vi "Autonomous Independent.vi"() -> ()   [LabVIEW 2013]
doc: "This VI is called when autonomous begins, and will automatically be terminated when autonomous ends. You can carry out timed or sensor driven robot movement independently without needing to return to the caller."
uses:
  Autonomous Setpoints.ctl
  Autonomous Center Line Setpoints.ctl
  Autonomous Commands.ctl
  Robot Global Data.vi
  <vilib>/Rock Robotics/WPI/RobotDrive/WPI_RobotDriveGetSetRefNum.vi
  <vilib>/Rock Robotics/WPI/RobotDrive/WPI_RobotDriveArcadeDrive_Standard(NoSaturation).vi
  <vilib>/addons/control/pid/pid.llb/PID (DBL).vi
  <vilib>/Rock Robotics/WPI/Joystick/WPI_JoystickGetSetRefNum.vi
  <vilib>/addons/control/pid/NI_PID_pid.lvlib
panel:
  out "Distance PID":T1
  out "Auto-Center Line":T2={"Arc Turn x-axis"=0.0, "Arc Turn y-axis"=0.8999999999999999, "Arc Turn Distance"=6.0, "Distance 1"=11.0, "Two Disc Distance 1"=0.0, "Distance 2"=-2.0, "Two Disc Distance 2"=0.0, "Spin Angle"=-70.0, "Spin Angle tolerance"=5.0, "Spin y-axis"=0.0, "Spin Distance"=0.0, "Center Line Enabled"=FALSE, "Distance 3"=8.5, "Two Disc Distance 3"=0.0, "Spin Angle 2"=90.0, "Spin Angle tolerance 2"=15.0, "Spin y-axis 2"=0.0, "Spin Distance 2"=0.0, "Shoot Angle 1"=14.6, "Disc Count 1"=4.0, "Shoot Time 1"=8000.0, "Shoot Angle 3"=16.4, "Disc Count 3"=5.0, "Shoot Time 3"=15000.0, "Low Gear"=TRUE}
  out "Auto Setpoints":T3={"Shoot Angle 1"=24.5, "Initial Delay"=0.0, "Disc Count 1"=3.0, "Shoot Time 1"=6000.0, "Distance 1"=6.5, "Two Disc Distance 1"=3.5, "Distance 2"=7.5, "Two Disc Distance 2"=3.5, "Distance 3"=-7.0, "Two Disc Distance 3"=0.0, "Shoot Angle 3"=31.0, "Disc Count 3"=4.0, "Shoot Time 3"=15000.0, "Distance 4"=0.0, "Two Disc Distance 4"=0.0, "Low Gear"=TRUE, "Shoot 1 Post Delay"=500.0}
  in  "Shoot Time 2":dbl
  in  "Disc Count 2":dbl
  in  "Shoot Angle 2":dbl
  out "Right Encoder":dbl(graph)
  out "Left Encoder":dbl(graph)
  out "Y axis Speed":dbl(graph)
  out "Steering":dbl(graph)
  out "Current Movement, for debugging":T4 {"Y Joystick Value" scale=1.0..-1.0; "X Joystick Value" scale=-1.0..1.0}
  in  "Array of robot movements":T5(array[cluster]) {"Y Joystick Value" scale=1.0..-1.0; "X Joystick Value" scale=-1.0..1.0}
  # "Be sure to right-click and choose Data Operations>>Make Current Value default if you want to save the array values with the VI"
  # "SKIP"
  # "SKIP"
  # "(Shoot 2 is not run)"
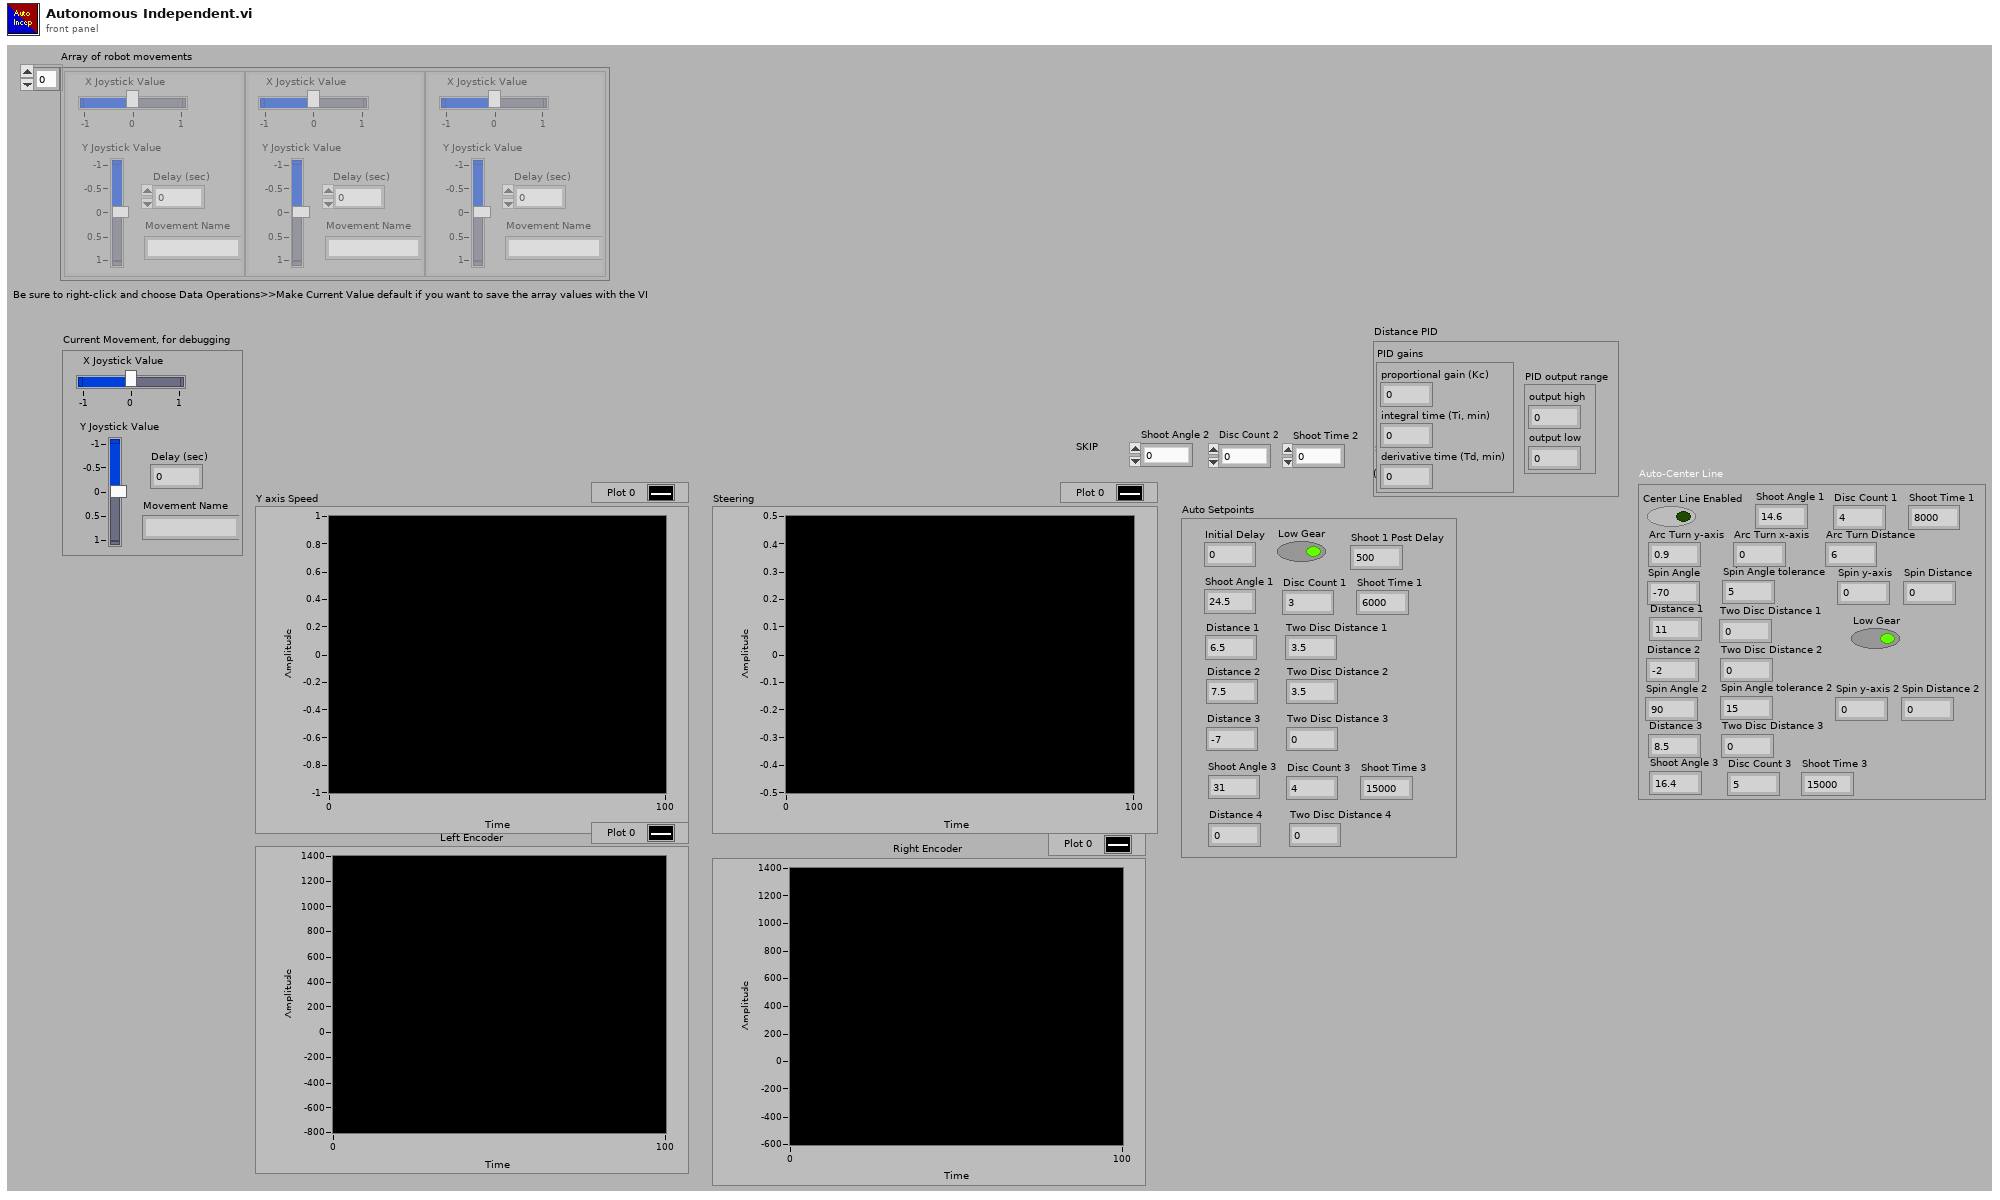
[diagram p1: front panel]
types:
  T1 = cluster{"PID gains":cluster{"proportional gain (Kc)":dbl, "integral time (Ti, min)":dbl, "derivative time (Td, min)":dbl}, "PID output range":cluster{"output high":dbl, "output low":dbl}}
  T2 = typedef "Autonomous Center Line Setpoints.ctl" = cluster{"Arc Turn x-axis":dbl, "Arc Turn y-axis":dbl, "Arc Turn Distance":dbl, "Distance 1":dbl, "Two Disc Distance 1":dbl, "Distance 2":dbl, "Two Disc Distance 2":dbl, "Spin Angle":dbl, "Spin Angle tolerance":dbl, "Spin y-axis":dbl, "Spin Distance":dbl, "Center Line Enabled":bool, "Distance 3":dbl, "Two Disc Distance 3":dbl, "Spin Angle 2":dbl, "Spin Angle tolerance 2":dbl, "Spin y-axis 2":dbl, "Spin Distance 2":dbl, "Shoot Angle 1":dbl, "Disc Count 1":dbl, "Shoot Time 1":dbl, "Shoot Angle 3":dbl, "Disc Count 3":dbl, "Shoot Time 3":dbl, "Low Gear":bool}
  T3 = typedef "Autonomous Setpoints.ctl" = cluster{"Shoot Angle 1":dbl, "Initial Delay":dbl, "Disc Count 1":dbl, "Shoot Time 1":dbl, "Distance 1":dbl, "Two Disc Distance 1":dbl, "Distance 2":dbl, "Two Disc Distance 2":dbl, "Distance 3":dbl, "Two Disc Distance 3":dbl, "Shoot Angle 3":dbl, "Disc Count 3":dbl, "Shoot Time 3":dbl, "Distance 4":dbl, "Two Disc Distance 4":dbl, "Low Gear":bool, "Shoot 1 Post Delay":dbl}
  T4 = cluster{"X Joystick Value":dbl, "Y Joystick Value":dbl, "Delay (sec)":dbl, "Movement Name":string}
  T5 = cluster{"X Joystick Value":dbl, "Y Joystick Value":dbl, "Delay (sec)":dbl, "Movement Name":string}[]
  T6 = typedef "Autonomous Commands.ctl" = cluster{"Load":bool, "Warmup":bool, "Low Gear":bool, "Shoot Angle":dbl, "Azimuth":bool, "Elevator":bool, "Neutral Angle":dbl, "Two Discs":bool, "Shoot":bool}
  T7 = typedef "WPI_RobotDriveDevRef.ctl" = cluster{"DevStatus":errorcluster, "Motors[]":T8[], "Square Inputs":bool, "Max Output":dbl, "Isochronous":bool}
  T8 = typedef "WPI_MotorControlDeviceRef.ctl" = cluster{"DeviceStatus":errorcluster, "Type":enum16{"PWM", "CAN"}, "PWM":cluster{"Digital Module":T9, "PWM Channel":T10, "DeadBand":T11}, "CAN":cluster{"Device Number":u8, "Control Mode":T12, "Semaphore":T13, "Max Vout":dbl}, "Invert":bool, "TransformRef":T14, "InvTransformRef":T14}
  T9 = typedef "FPGA_TypedefDigitalModule.ctl" = enum16{"Digital Module 1", "Digital Module 2"}
  T10 = typedef "FPGA_DIOPWMChannel.ctl" = enum8{"PWM 1", "PWM 2", "PWM 3", "PWM 4", "PWM 5", "PWM 6", "PWM 7", "PWM 8", "PWM 9", "PWM 10", "Invalid"}
  T11 = typedef "WPI_PWMDeadband.ctl" = cluster{"Name":string, "maxPositivePwm":i32, "minPositivePwm":i32, "centerPwm":i32, "maxNegativePwm":i32, "minNegativePwm":i32, "angularRange":u16}
  T12 = typedef "WPI_CANJaguar_ControlMode.ctl" = enum8{"Percent VBus", "Current", "Speed", "Position", "Voltage"}
  T13 = typedef "Semaphore RefNum" = refnum<k1>
  T14 = typedef "WPI_PWMTransform_ConPane.ctl" = refnum<vi>
  T15 = typedef "UDP Dashboard Packet.ctl" = cluster{"Feed Angle":dbl, "Neutral Angle":dbl, "Autonomous Setpoints":T3, "Auto Shift":T16, "Elevator Angle Offset":dbl, "Potentiometer Angle":cluster{"Pot M":dbl, "Pot B":dbl}, "Shoot Setpoints":cluster{"Vision":T17, "Back Corner":T17, "Front":T17, "Front Corner":T17, "Half Court":T17, "Full Court":T17, "Pyramid":T17}, "Halo Drive":T18, "Auto Speed Constants":T19, "Shooting Delays":cluster{"Unjam On":dbl, "Unjam Off":dbl, "Flipper On":dbl, "Flipper Off":dbl, "Hopper Up":dbl}, "Left Roller Pwr":dbl, "Right Roller Pwr":dbl, "Elevator PID Gains":cluster{"proportional gain (Kc)":dbl, "integral time (Ti, min)":dbl, "derivative time (Td, min)":dbl}, "Elevator PID Output Range":cluster{"output high":dbl, "output low":dbl}, "Elevator Angle Tolerance":dbl, "Toggle Ears Delay":dbl, "Toggle Ears Distance":dbl, "Unjam Servo Angle":dbl, "Auton Steer PID gains":cluster{"proportional gain (Kc)":dbl, "integral time (Ti, min)":dbl, "derivative time (Td, min)":dbl}, "Auton Steer output range":cluster{"output high":dbl, "output low":dbl}, "Auto Reverse Speed":dbl, "Auto Stop Throttle":dbl, "Auto Stop Duration":dbl, "Spin output range":cluster{"output high":dbl, "output low":dbl}, "Spin PID gains":cluster{"proportional gain (Kc)":dbl, "integral time (Ti, min)":dbl, "derivative time (Td, min)":dbl}, "Auto-Center Line":T2, "Auton Distance PID gains Low Gear":cluster{"proportional gain (Kc)":dbl, "integral time (Ti, min)":dbl, "derivative time (Td, min)":dbl}, "Auton Distance output range":cluster{"output high":dbl, "output low":dbl}, "Auton Distance Threshold":dbl, "Auton Velocity Cutoff":dbl, "Auton Distance output range Center Line":cluster{"output high":dbl, "output low":dbl}, "Auton Distance PID gains High Gear":cluster{"proportional gain (Kc)":dbl, "integral time (Ti, min)":dbl, "derivative time (Td, min)":dbl}}
  T16 = typedef "Auto Shift Settings.ctl" = cluster{"Enabled":bool, "Upshift Speed":dbl, "Downshift Speed":dbl, "Upshift Throttle":dbl, "Turn Power Diff":dbl, "Motor Limit":dbl, "Encoder Limit":dbl}
  T17 = typedef "Shoot Profile.ctl" = cluster{"Pre RPM":dbl, "Main RPM":dbl, "Angle":dbl}
  T18 = typedef "Halo Drive.ctl" = cluster{"Gains":cluster{"Quickturn_Sens_Low":dbl, "Quickturn_Sens_High":dbl, "Speedturn_Sens_Low":dbl, "Speedturn_Sens_High":dbl}, "QuickTurn Const":dbl, "Loading Throttle Limit":dbl}
  T19 = typedef "Auto Speed Constants.ctl" = cluster{"Slowing Distance":dbl, "High Speed":dbl, "Rampup Time":dbl, "Low Speed":dbl, "High Speed (Reverse)":dbl}
  T20 = cluster{"proportional gain (Kc)":dbl, "integral time (Ti, min)":dbl, "derivative time (Td, min)":dbl}
  T21 = typedef "WPI_GyroDevRef.ctl" = cluster{"DevStatus":errorcluster, "Analog Module":T22, "Analog Channel":T23, "Offset":dbl, "Gain (VoltsPerDegree/Second)":dbl}
  T22 = typedef "FPGA_TypedefAnalogModule.ctl" = enum16{"Analog Module 1", "Analog Module 2"}
  T23 = typedef "FPGA_AIChannel.ctl" = enum8{"AI 1", "AI 2", "AI 3", "AI 4", "AI 5", "AI 6", "AI 7", "AI 8", "Invalid"}
  T24 = typedef "WPI_JoystickDevRef.ctl" = cluster{"Device":T25}
  T25 = typedef "WPI_JoystickDeviceEnum.ctl" = enum16{"USB 1", "USB 2", "USB 3", "USB 4", "Kinect 1", "Kinect 2"}
  T26 = cluster{"axis 1 (x)":dbl, "axis 2 (y)":dbl, "axis 3 (throttle)":dbl, "axis 4":dbl, "axis 5":dbl, "axis 6":dbl}
  T27 = typedef "WPI_EncoderDevRef.ctl" = cluster{"DevStatus":errorcluster, "EncoderIndex":T28, "CounterIndex":T29, "DistancePerCount":dbl, "Decoding Type":T30}
  T28 = typedef "FPGA_EncoderIdx.ctl" = enum8{"Enc 0", "Enc 1", "Enc 2", "Enc 3", "Invalid"}
  T29 = typedef "FPGA_CounterCtrSystemIndex.ctl" = enum8{"Ctr 0", "Ctr 1", "Ctr 2", "Ctr 3", "Ctr 4", "Ctr 5", "Ctr 6", "Ctr 7", "Invalid"}
  T30 = typedef "WPI_EncoderType.ctl" = enum16{"1x", "2x", "4x"}
  T31 = typedef "Encoder Values.ctl" = cluster{"Left Dist":dbl, "Left Speed":dbl, "Right Dist":dbl, "Right Speed":dbl, "Left Ticks":dbl, "Right Ticks":dbl, "Avg Distance":dbl, "Avg Speed":dbl}
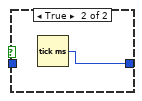
[diagram p3: hidden frame]
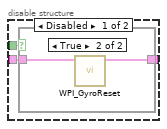
[diagram p4: hidden frame]
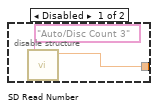
[diagram p6: hidden frame]
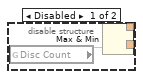
[diagram p7: hidden frame]
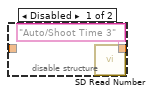
[diagram p8: hidden frame]
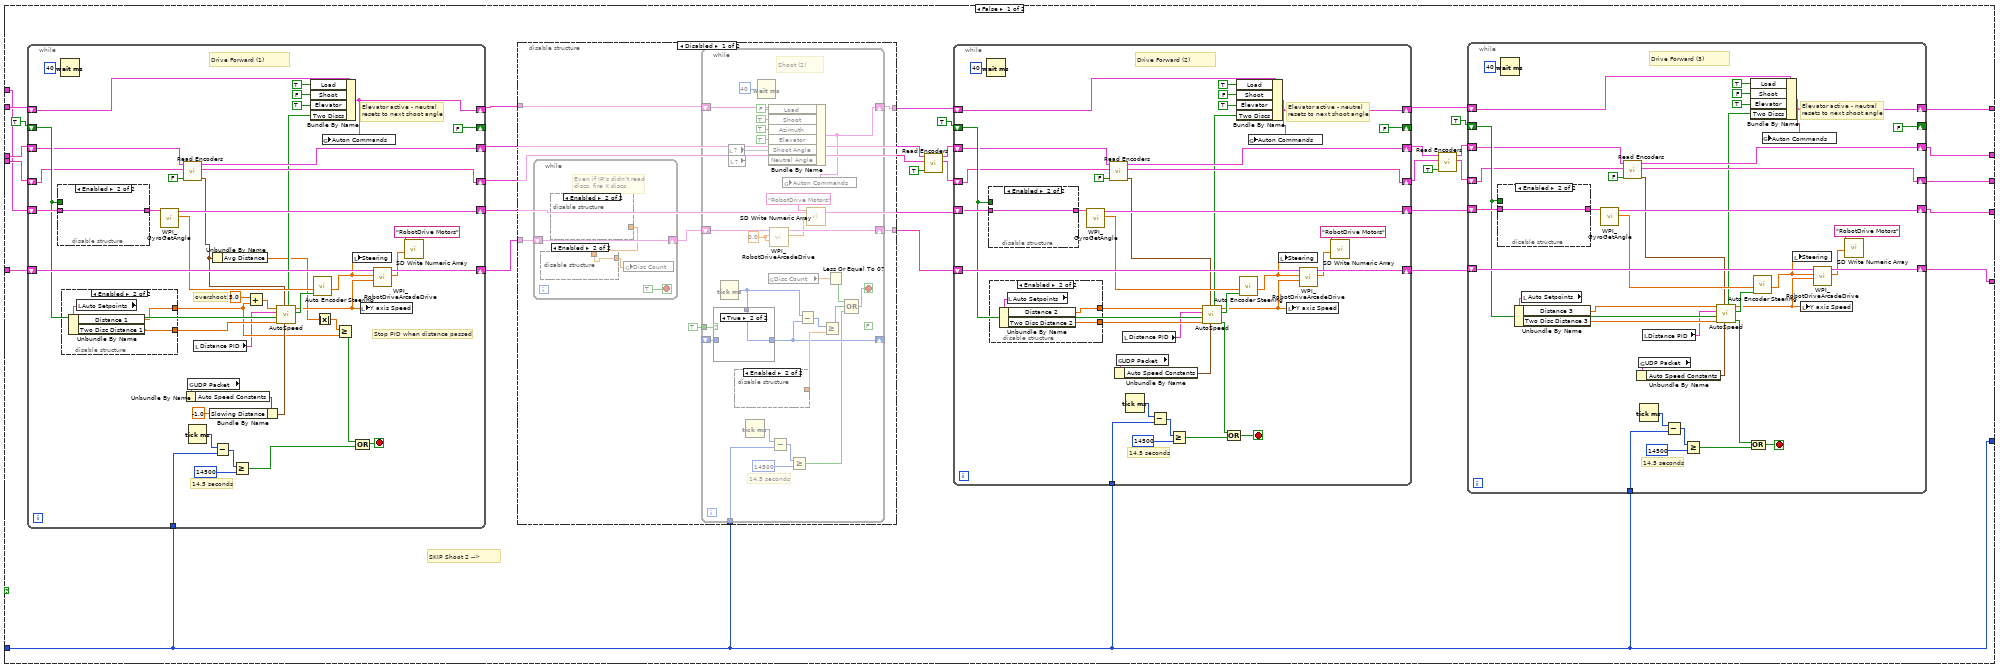
[diagram p10: hidden frame]
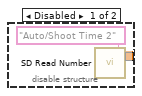
[diagram p11: hidden frame]
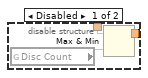
[diagram p13: hidden frame]
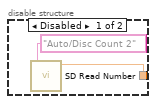
[diagram p14: hidden frame]
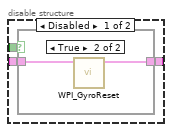
[diagram p16: hidden frame]
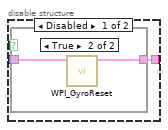
[diagram p18: hidden frame]
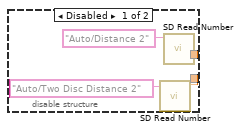
[diagram p20: hidden frame]
diagram:
  (unwired) "This code sets the toggle rate used by the Periodic Tasks VI.  For autonomous mode we slowly flash the USER1 LED on the cRIO.  Look at the Periodic Tasks VI to see how this global value is used."
  (unwired) "Autonomous sample code is disabled so your robot doesn't unexpectantly run in Autonomous mode.  To enable this code, right-click on the edge of the frame and choose either \"Remove Diagram Disable Structure\" or \"Enable This Subdiagram\". You should only enable one of the samples."
  (unwired) "This function is run in parallel when the autonomous period begins. It will be terminated automatically when the period ends.\n\nNote that all Driver Station inputs are automatically latched and will not change once auto begins."
  # "SKIP Shoot 2 -->"
  # "Every 20ms, report that we are running autonomous\ncode. Loop will abort the same time as the VI."
  # "Auton\nstart time"
  # "Auto\n\nShoot 3\n\nGo forward\nPick up center pyramid discs\nShoot 2\n\n\nPick up front pyramid discs\nGo back\nShoot 2"
  # "This gives you the joystick value\nthat is often the throttle"
  # "Use time and/or sensors to control how the robot drives."
  # "This tells you the driver position\nand alliance color"
  # "This gives you the eight Driver Station\ndigital switch settings"
  # "This gives you the four\nDriver Station sliders or\nanalog voltages"
  n1 = call <vilib>:"WPI_RobotDriveRefNum Registry Get.vi"("refnum name"="Left and Right Motors") -> ("RobotDriveDevRef"=w15:T7)  [unwired: 1 in, 9 out]
  n2 = while {
    tunnel: w15 -> [w47]
    tunnel: [w47] -> w14
    tunnel: [w44] -> w12
    tunnel: [w25] -> w4
    stop <- TRUE stop-if-true
    # "Replace Shoot 1 and 3 controls\nif in Center Line mode"
    n3 = global read "Robot Global Data.vi" "UDP Packet"() -> (w45:T15)
    n4 = Unbundle By Name(w45) -> ("Auton Distance PID gains Low Gear"=w30:T20, "Auton Distance PID gains High Gear"=w29:T20, "Auton Distance output range Center Line"=w26:cluster{"output high":dbl, "output low":dbl}, "Auton Distance output range"=w24:cluster{"output high":dbl, "output low":dbl}, "Autonomous Setpoints"=w43:T3, "Auto-Center Line"=w33:T2)
    "Auto-Center Line" <- w33
    n5 = Unbundle By Name(w33) -> ("Center Line Enabled"=w25:bool, "Shoot Angle 1"=w37:dbl, "Disc Count 1"=w38:dbl, "Shoot Time 1"=w39:dbl, "Shoot Angle 3"=w40:dbl, "Disc Count 3"=w41:dbl, "Shoot Time 3"=w42:dbl, "Low Gear"=w34:bool)
    n6 = Tick Count (ms)() -> (millisecond timer value=w44:u32)
    n7 = global write "Robot Global Data.vi" "Azimuth Ready"(TRUE ("Azimuth Ready")) -> ()
    n8 = case shown="True" w25 {
      tunnel: w43 -> [w49 w58]
      tunnel: [w49 w57] -> w32
      tunnel: w42 -> [_ w56]
      tunnel: w41 -> [_ w55]
      tunnel: w40 -> [_ w54]
      tunnel: w39 -> [_ w53]
      tunnel: w38 -> [_ w52]
      tunnel: w37 -> [_ w51]
      tunnel: w34 -> [_ w50]
      frame False {
      }
      frame True {
        n9 = Bundle By Name(cluster=w58, "Shoot Angle 1"=w51, "Disc Count 1"=w52, "Shoot Time 1"=w53, "Shoot Angle 3"=w54, "Disc Count 3"=w55, "Shoot Time 3"=w56, "Low Gear"=w50) -> (w57:T3)
      }
    }
    "Auto Setpoints" <- w32
    n10 = Unbundle By Name(w32) -> ("Low Gear"=w31:bool)
    n11 = Select(t=w30, s=w31, f=w29) -> (s? t:f=w28:T20)
    n12 = Select(t=w26, s=w25, f=w24) -> (s? t:f=w27:cluster{"output high":dbl, "output low":dbl})
    n13 = Bundle By Name(cluster=T1 {"PID gains"={"proportional gain (Kc)"=0.0, "integral time (Ti, min)"=0.0, "derivative time (Td, min)"=0.0}, "PID output range"={"output high"=0.0, "output low"=0.0}} ("Distance PID"), "PID gains"=w28, "PID output range"=w27) -> (→"Distance PID":T1)
  }
  n14 = while {
    stop <- FALSE stop-if-true
    n15 = call <vilib>:"WPI_DriverStationReport Robot Code State.vi"("Autonomous"=TRUE) -> ()  [unwired: 10 in, 1 out]
    n16 = Wait (ms)(milliseconds to wait=u32 20) -> ()  [unwired: 1 out]
  }
  n17 = disable-structure shown="Disabled" {
    frame Disabled {
      n18 = call <vilib>:"SD Read Number.vi"("Name"="Auto/Shoot Angle 1") -> ()  [unwired: 8 in, 3 out]
      n19 = call <vilib>:"SD Read Number.vi"("Name"="Auto/Shoot Angle 2") -> ()  [unwired: 8 in, 3 out]
      n20 = call <vilib>:"SD Read Number.vi"("Name"="Auto/Shoot Angle 3") -> ()  [unwired: 8 in, 3 out]
    }
    frame Enabled {
    }
  }
  n21 = global write "Robot Global Data.vi" "LED toggle rate (ms)"(u32 500 ("LED ms toggle rate")) -> ()
  n22 = disable-structure shown="Enabled" {
    frame Disabled {
      n23 = call <vilib>:"SD Read Boolean.vi"("Name"="Auto/Low Gear") -> ()  [unwired: 8 in, 3 out]
    }
    frame Enabled {
    }
  }
  n24 = while {
    tunnel: w14 -> [_]
    stop <- FALSE stop-if-true
    n25 = Wait (ms)(milliseconds to wait=u32 90) -> ()  [unwired: 1 out]
    n26 = call "Motor Output Report.vi"("Motor Speed"=0.0, "Motor refnum name"="Lift Motor 1" ("refnum name")) -> ()  [unwired: 9 in, 1 out]
  }
  n27 = call <vilib>:"WPI_DriverStationGet Alliance Info.vi"() -> ()  [unwired: 12 out]
  n28 = call <vilib>:"WPI_DriverStationGet Analog Input.vi"() -> ()  [unwired: 12 out]
  n29 = call <vilib>:"WPI_DriverStationGet Digital Input.vi"() -> ("Driver Station Digital Input (1-8)"=w23:bool[])  [unwired: 11 out]
  n30 = call <vilib>:"WPI_GyroRefNum Registry Get.vi"("refnum name"="Gyro") -> ("GyroDevRef"=w6:T21)  [unwired: 9 in, 1 out]
  n31 = while {
    shift-right: [w103] -> w11
    shift-left: w14 -> [w103]
    shift-right: [w100] -> _
    shift-left: _ -> [w99]
    shift-right: [FALSE] -> _
    shift-left: TRUE -> [w98]
    shift-right: [w95] -> w9
    shift-left: T6 {"Load"=FALSE, "Warmup"=FALSE, "Low Gear"=FALSE, "Shoot Angle"=35.0, "Azimuth"=FALSE, "Elevator"=FALSE, "Neutral Angle"=0.0, "Two Discs"=FALSE, "Shoot"=FALSE} ("Auton Commands") -> [w94]
    tunnel: w12 -> [w75]
    shift-right: [FALSE ("Load")] -> _
    shift-left: TRUE ("Elevator") -> [w74]
    shift-right: [w71] -> w5
    shift-left: w6 -> [w72]
    stop <- w77 stop-if-true
    # "14.5 seconds"
    # "Delay"
    # "Start with 3 Discs"
    n32 = local read "Auto Setpoints"() -> (w88:T3)
    n33 = Unbundle By Name(w88) -> ("Low Gear"=w85:bool, "Shoot Angle 1"=w87:dbl, "Shoot Angle 3"=w86:dbl, "Disc Count 1"=w84:dbl, "Initial Delay"=w82:dbl)
    n34 = case shown="True" w74 {
      tunnel: w72 -> [w104 w106]
      tunnel: [w104 w105] -> w71
      frame False {
      }
      frame True {
        n35 = call <vilib>:"WPI_GyroReset.vi"("GyroDevRef"=w106) -> ("GyroDevRef"=w105:T21)  [unwired: 9 in, 1 out]
      }
    }
    n36 = disable-structure shown="Enabled" {
      disable-tunnel: [w108 w109] -> w102
      disable-tunnel: w84 -> [_ w109]
      frame Disabled {
        n37 = call <vilib>:"SD Read Number.vi"("Name"="Auto/Disc Count 1") -> ("Numeric"=w108:dbl)  [unwired: 8 in, 2 out]
      }
      frame Enabled {
      }
    }
    n38 = Tick Count (ms)() -> (millisecond timer value=w96:u32)
    n39 = case shown="False" w98 {
      tunnel: [w113 w114] -> w100
      tunnel: w99 -> [w113 _]
      tunnel: w96 -> [_ w114]
      frame False {
      }
      frame True {
      }
    }
    n40 = disable-structure shown="Enabled" {
      disable-tunnel: [w110 w112] -> w83
      disable-tunnel: w82 -> [_ w112]
      frame Disabled {
        n41 = call <vilib>:"SD Read Number.vi"("Name"="Auto/Initial Delay") -> ("Numeric"=w110:dbl)  [unwired: 8 in, 2 out]
      }
      frame Enabled {
      }
    }
    n42 = Tick Count (ms)() -> (millisecond timer value=w81:u32)
    n43 = Subtract(x=w81, y=w75) -> (x-y=w80:u32)
    n44 = Greater Or Equal?(x=w80, y=u32 14500) -> (x >= y?=w76:bool)
    n45 = Bundle By Name(cluster=w94, "Load"=FALSE, "Shoot"=FALSE, "Low Gear"=w85, "Shoot Angle"=w87, "Azimuth"=FALSE, "Elevator"=TRUE, "Neutral Angle"=w86, "Two Discs"=FALSE, "Warmup"=FALSE) -> (w95:T6)
    n46 = global write "Robot Global Data.vi" "Auton Commands"(w95) -> ()
    n47 = Subtract(x=w96, y=w100) -> (x-y=w101:u32)
    n48 = global write "Robot Global Data.vi" "Disc Count"(w102) -> ()
    n49 = Greater Or Equal?(x=w101, y=w83) -> (x >= y?=w78:bool)
    n50 = Compound Arithmetic op=OR(w78, w76) -> (w77:bool)
  }
  n51 = call <vilib>:"WPI_JoystickRefNum Registry Get.vi"("refnum name"="Joystick 1") -> ("JoystickDevRef"=w21:T24)  [unwired: 1 in, 9 out]
  n52 = call <vilib>:"WPI_JoystickGet.vi"("JoystickDevRef"=w21) -> ("Axes"=w18:T26)  [unwired: 1 in, 5 out]
  n53 = Cluster To Array(cluster=w18) -> (array=w19:dbl[])
  n54 = Unbundle By Name(w18) -> ()  [unwired: 1 out]
  n55 = call <vilib>:"SD Write Numeric Array.vi"("Numeric Array"=w19, "Name"="Joystick 1/Axes") -> ()  [unwired: 8 in, 2 out]
  n56 = Index Array(array=w23) -> (element #1=w1:bool)  [unwired: 8 in, 7 out]
  n57 = disable-structure shown="Disabled" {
    frame Disabled {
      w115 = "RobotDrive Motors" ("Name")
      # "This is some simple sample code to drive your robot curving one direction and then the other."
      # "stand still"
      # "turn left for 0.5 second"
      # "turn right for 1 second"
      n58 = call <vilib>:"WPI_RobotDriveRefNum Registry Get.vi"("refnum name"="Left and Right Motors") -> ("RobotDriveDevRef"=w119:T7)  [unwired: 1 in, 9 out]
      n59 = call-poly <vilib>:"WPI_RobotDriveArcadeDrive.vi"("Y axis value"=0.5 ("X axis value"), "X axis value"=0.25, "RobotDriveDevRef"=w119) -> ("Motor Values"=w118:dbl[], "RobotDriveDevRef"=w126:T7)  [unwired: 1 in, 6 out]
      n60 = call <vilib>:"SD Write Numeric Array.vi"("Numeric Array"=w118, "Name"=w115) -> ()  [unwired: 8 in, 2 out]
      n61 = call <vilib>:"WPI_RobotDriveDelayAndUpdateSafety.vi"("Delay (s)"=1.0, "RobotDriveDevRef"=w126) -> ("RobotDriveDevRef 2"=w125:T7)  [unwired: 8 in, 1 out]
      n62 = call-poly <vilib>:"WPI_RobotDriveArcadeDrive.vi"("Y axis value"=0.25 ("X axis value"), "X axis value"=0.5, "RobotDriveDevRef"=w125) -> ("Motor Values"=w117:dbl[], "RobotDriveDevRef"=w124:T7)  [unwired: 1 in, 6 out]
      n63 = call <vilib>:"SD Write Numeric Array.vi"("Numeric Array"=w117, "Name"=w115) -> ()  [unwired: 8 in, 2 out]
      n64 = call <vilib>:"WPI_RobotDriveDelayAndUpdateSafety.vi"("Delay (s)"=0.5, "RobotDriveDevRef"=w124) -> ("RobotDriveDevRef 2"=w123:T7)  [unwired: 8 in, 1 out]
      n65 = call-poly <vilib>:"WPI_RobotDriveArcadeDrive.vi"("Y axis value"=0.0 ("X axis value"), "X axis value"=0.0, "RobotDriveDevRef"=w123) -> ("Motor Values"=w116:dbl[])  [unwired: 1 in, 7 out]
      n66 = call <vilib>:"SD Write Numeric Array.vi"("Numeric Array"=w116, "Name"=w115) -> ()  [unwired: 8 in, 2 out]
    }
    frame Enabled {
    }
  }
  n67 = disable-structure shown="Disabled" {
    frame Disabled {
      # "This sample code describes robot movements in an array. You can extend it to control other motors\non your robot. You can also use file I/O to move the data to a text file."
      n68 = call <vilib>:"WPI_RobotDriveRefNum Registry Get.vi"("refnum name"="Left and Right Motors") -> ("RobotDriveDevRef"=w134:T7)  [unwired: 1 in, 9 out]
      n69 = for {
        shift-right: [w140] -> _
        shift-left: w134 -> [w141]
        tunnel: "Array of robot movements" -> [w136] mode=indexing
        n70 = Unbundle By Name(w136) -> ("X Joystick Value"=w139:dbl, "Y Joystick Value"=w138:dbl, "Delay (sec)"=w137:dbl)  [unwired: 1 out]
        n71 = call-poly <vilib>:"WPI_RobotDriveArcadeDrive.vi"("Y axis value"=w138, "X axis value"=w139, "RobotDriveDevRef"=w141) -> ("Motor Values"=w143:dbl[], "RobotDriveDevRef"=w142:T7)  [unwired: 1 in, 6 out]
        n72 = call <vilib>:"SD Write Numeric Array.vi"("Numeric Array"=w143, "Name"="RobotDrive Motors") -> ()  [unwired: 8 in, 2 out]
        n73 = call <vilib>:"WPI_RobotDriveDelayAndUpdateSafety.vi"("Delay (s)"=w137, "RobotDriveDevRef"=w142) -> ("RobotDriveDevRef 2"=w140:T7)  [unwired: 8 in, 1 out]
        "Current Movement, for debugging" <- w136
      }
    }
    frame Enabled {
    }
  }
  n74 = case shown="False" w1 {
    tunnel: w12 -> [w146 w887]
    tunnel: w11 -> [w178 w906]
    tunnel: w9 -> [w175 w898]
    tunnel: w5 -> [w169 w897]
    tunnel: w4 -> [w154 _]
    tunnel: [w150 w892] -> w3
    tunnel: [w149 w893] -> w2
    frame False {
      # "Stop from coasting backwards"
      # "SKIP Shoot 2 -->"
      n75 = while {
        shift-right: [w873] -> w148
        shift-left: w178 -> [w874]
        shift-right: [w862] -> w177
        shift-left: w175 -> [w863]
        shift-right: [FALSE] -> _
        shift-left: TRUE -> [w857]
        shift-right: [w858] -> _
        shift-left: _ -> [w859]
        tunnel: w146 -> [w846]
        shift-right: [w842] -> w168
        shift-left: w169 -> [w842]
        stop <- w843 stop-if-true
        w871 = 0.0 ("Y axis value")
        # "14.5 seconds"
        # "Shoot (1)"
        n76 = local read "Auto Setpoints"() -> (w854:T3)
        n77 = Unbundle By Name(w854) -> ("Shoot Angle 1"=w853:dbl, "Shoot Angle 3"=w852:dbl, "Shoot Time 1"=w851:dbl)
        n78 = Tick Count (ms)() -> (millisecond timer value=w855:u32)
        n79 = case shown="True" w857 {
          tunnel: [w878 w879] -> w858
          tunnel: w859 -> [w878 _]
          tunnel: w855 -> [_ w879]
          frame False {
          }
          frame True {
          }
        }
        n80 = Wait (ms)(milliseconds to wait=u32 40) -> ()  [unwired: 1 out]
        n81 = disable-structure shown="Enabled" {
          disable-tunnel: [w875 w877] -> w856
          disable-tunnel: w851 -> [_ w877]
          frame Disabled {
            n82 = call <vilib>:"SD Read Number.vi"("Name"="Auto/Shoot Time 1") -> ("Numeric"=w875:dbl)  [unwired: 8 in, 2 out]
          }
          frame Enabled {
          }
        }
        n83 = Tick Count (ms)() -> (millisecond timer value=w847:u32)
        n84 = global read "Robot Global Data.vi" "Disc Count"() -> (w869:dbl)
        n85 = Subtract(x=w847, y=w846) -> (x-y=w848:u32)
        n86 = call-poly <vilib>:"WPI_RobotDriveArcadeDrive.vi"("Y axis value"=w871, "X axis value"=w871, "RobotDriveDevRef"=w874) -> ("Motor Values"=w872:dbl[], "RobotDriveDevRef"=w873:T7)  [unwired: 1 in, 6 out]
        n87 = Greater Or Equal?(x=w848, y=u32 14500) -> (x >= y?=w850:bool)
        n88 = Subtract(x=w855, y=w858) -> (x-y=w860:u32)
        n89 = call <vilib>:"SD Write Numeric Array.vi"("Numeric Array"=w872, "Name"="RobotDrive Motors") -> ()  [unwired: 8 in, 2 out]
        n90 = Bundle By Name(cluster=w863, "Load"=FALSE, "Shoot"=TRUE, "Azimuth"=FALSE, "Elevator"=TRUE, "Shoot Angle"=w853, "Neutral Angle"=w852) -> (w862:T6)
        n91 = global write "Robot Global Data.vi" "Auton Commands"(w862) -> ()
        n92 = Less Or Equal To 0?(x=w869) -> (x <= 0?=w844:bool)
        n93 = Greater Or Equal?(x=w860, y=w856) -> (x >= y?=w845:bool)
        n94 = Compound Arithmetic op=OR(w844, w845, w850) -> (w843:bool)
      }
      n95 = while {
        shift-right: [w196] -> w147
        shift-left: w148 -> [w197]
        tunnel: w146 -> [w190]
        shift-right: [FALSE] -> _
        shift-left: TRUE -> [w187]
        shift-right: [w185] -> _
        shift-left: _ -> [w184]
        stop <- w191 stop-if-true
        w198 = 0.0 ("Y axis value")
        # "Delay - after Shoot 1"
        # "14.5 seconds"
        n96 = local read "Auto Setpoints"() -> (w183:T3)
        n97 = Unbundle By Name(w183) -> ("Shoot 1 Post Delay"=w182:dbl)
        n98 = Tick Count (ms)() -> (millisecond timer value=w189:u32)
        n99 = case shown="True" w187 {
          tunnel: [w199 w200] -> w185
          tunnel: w184 -> [w199 _]
          tunnel: w189 -> [_ w200]
          frame False {
          }
          frame True {
          }
        }
        n100 = Tick Count (ms)() -> (millisecond timer value=w195:u32)
        n101 = Subtract(x=w195, y=w190) -> (x-y=w194:u32)
        n102 = Greater Or Equal?(x=w194, y=u32 14500) -> (x >= y?=w192:bool)
        n103 = Subtract(x=w189, y=w185) -> (x-y=w188:u32)
        n104 = Greater Or Equal?(x=w188, y=w182) -> (x >= y?=w181:bool)
        n105 = Compound Arithmetic op=OR(w181, w192) -> (w191:bool)
        n106 = call-poly <vilib>:"WPI_RobotDriveArcadeDrive.vi"("Y axis value"=w198, "X axis value"=w198, "RobotDriveDevRef"=w197) -> ("RobotDriveDevRef"=w196:T7)  [unwired: 1 in, 7 out]
      }
      n107 = call <vilib>:"WPI_EncoderRefNum Registry Get.vi"("refnum name"="Drive Encoder Left") -> ("EncoderDevRef"=w173:T27)  [unwired: 9 in, 1 out]
      n108 = call <vilib>:"WPI_EncoderRefNum Registry Get.vi"("refnum name"="Drive Encoder Right") -> ("EncoderDevRef"=w172:T27)  [unwired: 9 in, 1 out]
      n109 = call "Read Encoders.vi"("Reset"=TRUE, "Right Encoder"=w172, "Left Encoder"=w173) -> ("Right Encoder Out"=w170:T27, "Left Encoder Out"=w171:T27)  [unwired: 6 in, 1 out]
      n110 = case shown="True" w154 {
        tunnel: w146 -> [w310 w559]
        tunnel: w147 -> [w340 w605]
        tunnel: w177 -> [w339 w609]
        tunnel: w171 -> [w338 w608]
        tunnel: w170 -> [w337 w607]
        tunnel: w168 -> [w316 w606]
        tunnel: [w315 w576] -> w158
        tunnel: [w314 w575] -> w151
        tunnel: [w313 w574] -> w157
        tunnel: [w311 w572] -> w152
        tunnel: [w312 w573] -> w156
        tunnel: [w310 w559] -> w155
        frame False {
          # "SKIP Shoot 2 -->"
          n111 = while {
            shift-right: [w533] -> w320
            shift-left: w340 -> [w534]
            shift-right: [FALSE] -> _
            shift-left: TRUE -> [w518]
            shift-right: [w519] -> w318
            shift-left: w337 -> [w516]
            shift-right: [w520] -> w319
            shift-left: w338 -> [w517]
            shift-right: [w514] -> w317
            shift-left: w316 -> [w529]
            shift-right: [w521] -> w323
            shift-left: w339 -> [w522]
            tunnel: w310 -> [w505]
            stop <- w504 stop-if-true
            # "overshoot"
            # "Stop PID when distance passed"
            # "14.5 seconds"
            # "Elevator active - neutral\nresets to next shoot angle"
            # "Drive Forward (1)"
            n112 = disable-structure shown="Enabled" {
              disable-tunnel: w529 -> [w538 w542]
              disable-tunnel: w518 -> [w537 _]
              disable-tunnel: [w536 w542] -> w515
              frame Disabled {
                n113 = case shown="True" w537 {
                  tunnel: w538 -> [w539 w541]
                  tunnel: [w539 w540] -> w536
                  frame False {
                  }
                  frame True {
                    n114 = call <vilib>:"WPI_GyroReset.vi"("GyroDevRef"=w541) -> ("GyroDevRef"=w540:T21)  [unwired: 9 in, 1 out]
                  }
                }
              }
              frame Enabled {
              }
            }
            n115 = Wait (ms)(milliseconds to wait=u32 40) -> ()  [unwired: 1 out]
            n116 = disable-structure shown="Enabled" {
              disable-tunnel: [w545 w548] -> w496
              disable-tunnel: [w543 w547] -> w511
              frame Disabled {
                n117 = call <vilib>:"SD Read Number.vi"("Name"="Auto/Two Disc Distance 1") -> ("Numeric"=w543:dbl)  [unwired: 8 in, 2 out]
                n118 = call <vilib>:"SD Read Number.vi"("Name"="Auto/Distance 1") -> ("Numeric"=w545:dbl)  [unwired: 8 in, 2 out]
              }
              frame Enabled {
                n119 = local read "Auto Setpoints"() -> (w549:T3)
                n120 = Unbundle By Name(w549) -> ("Distance 1"=w548:dbl, "Two Disc Distance 1"=w547:dbl)
              }
            }
            n121 = call <vilib>:"WPI_GyroGetAngle.vi"("GyroDevRef"=w515) -> ("Angle"=w513:dbl, "GyroDevRef"=w514:T21)  [unwired: 7 in, 2 out]
            n122 = call "Read Encoders.vi"("Reset"=FALSE, "Right Encoder"=w516, "Left Encoder"=w517) -> ("Encoder Values"=w493:T31, "Right Encoder Out"=w519:T27, "Left Encoder Out"=w520:T27)  [unwired: 6 in]
            n123 = global read "Robot Global Data.vi" "UDP Packet"() -> (w503:T15)
            n124 = Unbundle By Name(w503) -> ("Auto Speed Constants"=w502:T19)
            n125 = Tick Count (ms)() -> (millisecond timer value=w506:u32)
            n126 = local read "Distance PID"() -> (w492:T1)
            n127 = Bundle By Name(cluster=w502, "Slowing Distance"=-1.0) -> (w500:T19)
            n128 = Unbundle By Name(w493) -> ("Avg Distance"=w494:dbl)
            n129 = Subtract(x=w506, y=w505) -> (x-y=w507:u32)
            n130 = Greater Or Equal?(x=w507, y=u32 14500) -> (x >= y?=w509:bool)
            n131 = Add(x=5.0, y=w496) -> (x+y=w498:dbl)
            n132 = call "AutoSpeed.vi"("Auto Speed Constants"=w500, "Encoder Values"=w493, "Two Disc Distance"=w511, "Reinitialize"=w518, "PID settings"=w492, "Target Distance"=w498) -> ("Backward"=w528:bool, "Y axis Speed"=w527:dbl, "Two Disc Loading"=w510:bool)  [unwired: 2 in, 1 out]
            n133 = Bundle By Name(cluster=w522, "Load"=TRUE, "Shoot"=FALSE, "Elevator"=TRUE, "Two Discs"=w510) -> (w521:T6)
            n134 = call "Auto Encoder Steering.vi"("Backward"=w528, "Gyro Angle"=w513) -> ("Steering"=w526:dbl)  [unwired: 8 in, 1 out]
            n135 = Absolute Value(x=w494) -> (abs(x)=w495:dbl)
            n136 = global write "Robot Global Data.vi" "Auton Commands"(w521) -> ()
            n137 = Greater Or Equal?(x=w495, y=w496) -> (x >= y?=w497:bool)
            n138 = local write "Steering"(w526) -> ()
            n139 = Compound Arithmetic op=OR(w497, w509) -> (w504:bool)
            n140 = local write "Y axis Speed"(w527) -> ()
            n141 = call-poly <vilib>:"WPI_RobotDriveArcadeDrive.vi"("Y axis value"=w527, "X axis value"=w526, "RobotDriveDevRef"=w534) -> ("Motor Values"=w532:dbl[], "RobotDriveDevRef"=w533:T7)  [unwired: 1 in, 6 out]
            n142 = call <vilib>:"SD Write Numeric Array.vi"("Numeric Array"=w532, "Name"="RobotDrive Motors") -> ()  [unwired: 8 in, 2 out]
          }
          n143 = disable-structure shown="Disabled" {
            disable-tunnel: w323 -> [w347 w393]
            disable-tunnel: [w346 w393] -> w322
            disable-tunnel: [w345 w392] -> w321
            disable-tunnel: w320 -> [w344 w392]
            disable-tunnel: w310 -> [w342 _]
            frame Disabled {
              n144 = while {
                shift-right: [w383] -> w348
                shift-left: w344 -> [w383]
                stop <- TRUE stop-if-true
                # "Even if IR's didn't read\ndiscs, fire X discs"
                n145 = disable-structure shown="Enabled" {
                  disable-tunnel: [w391 _] -> w382
                  frame Disabled {
                    n146 = call <vilib>:"SD Read Number.vi"("Name"="Auto/Disc Count 2") -> ("Numeric"=w391:dbl)  [unwired: 8 in, 2 out]
                  }
                  frame Enabled {
                  }
                }
                n147 = disable-structure shown="Enabled" {
                  disable-tunnel: [w387 w389] -> w384
                  disable-tunnel: w382 -> [w386 w389]
                  frame Disabled {
                    n148 = global read "Robot Global Data.vi" "Disc Count"() -> (w388:dbl)
                    n149 = Max & Min(x=w386, y=w388) -> (max(x,y)=w387:dbl)  [unwired: 1 out]
                  }
                  frame Enabled {
                  }
                }
                n150 = global write "Robot Global Data.vi" "Disc Count"(w384) -> ()
              }
              n151 = while {
                shift-right: [w376] -> w345
                shift-left: w348 -> [w377]
                shift-right: [w359] -> w346
                shift-left: w347 -> [w366]
                tunnel: TRUE -> [w363]
                shift-right: [w362] -> _
                shift-left: _ -> [w361]
                tunnel: w342 -> [w352]
                stop <- w349 stop-if-true
                (unwired) FALSE
                w374 = 0.0 ("Y axis value")
                # "14.5 seconds"
                # "Shoot (2)"
                n152 = Tick Count (ms)() -> (millisecond timer value=w360:u32)
                n153 = case shown="True" w363 {
                  tunnel: [w380 w381] -> w362
                  tunnel: w361 -> [w380 _]
                  tunnel: w360 -> [_ w381]
                  frame False {
                  }
                  frame True {
                  }
                }
                n154 = local read item#-1() -> (w358)
                n155 = local read item#-1() -> (w357)
                n156 = disable-structure shown="Enabled" {
                  disable-tunnel: [w378 _] -> w364
                  frame Disabled {
                    n157 = call <vilib>:"SD Read Number.vi"("Name"="Auto/Shoot Time 2") -> ("Numeric"=w378:dbl)  [unwired: 8 in, 2 out]
                  }
                  frame Enabled {
                  }
                }
                n158 = Tick Count (ms)() -> (millisecond timer value=w356:u32)
                n159 = Wait (ms)(milliseconds to wait=u32 40) -> ()  [unwired: 1 out]
                n160 = global read "Robot Global Data.vi" "Disc Count"() -> (w372:dbl)
                n161 = Bundle By Name(cluster=w366, "Load"=FALSE, "Shoot"=TRUE, "Azimuth"=TRUE, "Elevator"=TRUE, "Shoot Angle"=w358, "Neutral Angle"=w357) -> (w359:T6)
                n162 = call-poly <vilib>:"WPI_RobotDriveArcadeDrive.vi"("Y axis value"=w374, "X axis value"=w374, "RobotDriveDevRef"=w377) -> ("Motor Values"=w375:dbl[], "RobotDriveDevRef"=w376:T7)  [unwired: 1 in, 6 out]
                n163 = Subtract(x=w356, y=w352) -> (x-y=w355:u32)
                n164 = global write "Robot Global Data.vi" "Auton Commands"(w359) -> ()
                n165 = Greater Or Equal?(x=w355, y=u32 14500) -> (x >= y?=w353:bool)
                n166 = Subtract(x=w360, y=w362) -> (x-y=w365:u32)
                n167 = call <vilib>:"SD Write Numeric Array.vi"("Numeric Array"=w375, "Name"="RobotDrive Motors") -> ()  [unwired: 8 in, 2 out]
                n168 = Greater Or Equal?(x=w365, y=w364) -> (x >= y?=w351:bool)
                n169 = Less Or Equal To 0?(x=w372) -> (x <= 0?=w350:bool)
                n170 = Compound Arithmetic op=OR(w350, w351, w353) -> (w349:bool)
              }
            }
            frame Enabled {
            }
          }
          n171 = call "Read Encoders.vi"("Reset"=TRUE, "Right Encoder"=w318, "Left Encoder"=w319) -> ("Right Encoder Out"=w336:T27, "Left Encoder Out"=w335:T27)  [unwired: 6 in, 1 out]
          n172 = while {
            shift-right: [w475] -> w328
            shift-left: w321 -> [w476]
            shift-right: [FALSE] -> _
            shift-left: TRUE -> [w461]
            shift-right: [w462] -> w326
            shift-left: w336 -> [w459]
            shift-right: [w463] -> w325
            shift-left: w335 -> [w460]
            shift-right: [w457] -> w327
            shift-left: w317 -> [w471]
            shift-right: [w451] -> w324
            shift-left: w322 -> [w452]
            tunnel: w310 -> [w446]
            stop <- w444 stop-if-true
            # "14.5 seconds"
            # "Elevator active - neutral\nresets to next shoot angle"
            # "Drive Forward (2)"
            n173 = Wait (ms)(milliseconds to wait=u32 40) -> ()  [unwired: 1 out]
            n174 = disable-structure shown="Enabled" {
              disable-tunnel: w471 -> [w480 w484]
              disable-tunnel: w461 -> [w479 _]
              disable-tunnel: [w478 w484] -> w458
              frame Disabled {
                n175 = case shown="True" w479 {
                  tunnel: w480 -> [w481 w483]
                  tunnel: [w481 w482] -> w478
                  frame False {
                  }
                  frame True {
                    n176 = call <vilib>:"WPI_GyroReset.vi"("GyroDevRef"=w483) -> ("GyroDevRef"=w482:T21)  [unwired: 9 in, 1 out]
                  }
                }
              }
              frame Enabled {
              }
            }
            n177 = disable-structure shown="Enabled" {
              disable-tunnel: [w487 w490] -> w464
              disable-tunnel: [w485 w489] -> w454
              frame Disabled {
                n178 = call <vilib>:"SD Read Number.vi"("Name"="Auto/Two Disc Distance 2") -> ("Numeric"=w485:dbl)  [unwired: 8 in, 2 out]
                n179 = call <vilib>:"SD Read Number.vi"("Name"="Auto/Distance 2") -> ("Numeric"=w487:dbl)  [unwired: 8 in, 2 out]
              }
              frame Enabled {
                n180 = local read "Auto Setpoints"() -> (w491:T3)
                n181 = Unbundle By Name(w491) -> ("Distance 2"=w490:dbl, "Two Disc Distance 2"=w489:dbl)
              }
            }
            n182 = call <vilib>:"WPI_GyroGetAngle.vi"("GyroDevRef"=w458) -> ("Angle"=w456:dbl, "GyroDevRef"=w457:T21)  [unwired: 7 in, 2 out]
            n183 = call "Read Encoders.vi"("Reset"=FALSE, "Right Encoder"=w459, "Left Encoder"=w460) -> ("Encoder Values"=w441:T31, "Right Encoder Out"=w462:T27, "Left Encoder Out"=w463:T27)  [unwired: 6 in]
            n184 = global read "Robot Global Data.vi" "UDP Packet"() -> (w443:T15)
            n185 = Unbundle By Name(w443) -> ("Auto Speed Constants"=w442:T19)
            n186 = local read "Distance PID"() -> (w440:T1)
            n187 = Tick Count (ms)() -> (millisecond timer value=w450:u32)
            n188 = Subtract(x=w450, y=w446) -> (x-y=w449:u32)
            n189 = Greater Or Equal?(x=w449, y=u32 14500) -> (x >= y?=w447:bool)
            n190 = call "AutoSpeed.vi"("Auto Speed Constants"=w442, "Encoder Values"=w441, "Two Disc Distance"=w454, "Reinitialize"=w461, "PID settings"=w440, "Target Distance"=w464) -> ("Finish"=w445:bool, "Backward"=w470:bool, "Y axis Speed"=w469:dbl, "Two Disc Loading"=w453:bool)  [unwired: 2 in]
            n191 = Compound Arithmetic op=OR(w445, w447) -> (w444:bool)
            n192 = Bundle By Name(cluster=w452, "Load"=TRUE, "Shoot"=FALSE, "Elevator"=TRUE, "Two Discs"=w453) -> (w451:T6)
            n193 = call "Auto Encoder Steering.vi"("Backward"=w470, "Gyro Angle"=w456) -> ("Steering"=w468:dbl)  [unwired: 8 in, 1 out]
            n194 = global write "Robot Global Data.vi" "Auton Commands"(w451) -> ()
            n195 = local write "Steering"(w468) -> ()
            n196 = local write "Y axis Speed"(w469) -> ()
            n197 = call-poly <vilib>:"WPI_RobotDriveArcadeDrive.vi"("Y axis value"=w469, "X axis value"=w468, "RobotDriveDevRef"=w476) -> ("Motor Values"=w474:dbl[], "RobotDriveDevRef"=w475:T7)  [unwired: 1 in, 6 out]
            n198 = call <vilib>:"SD Write Numeric Array.vi"("Numeric Array"=w474, "Name"="RobotDrive Motors") -> ()  [unwired: 8 in, 2 out]
          }
          n199 = call "Read Encoders.vi"("Reset"=TRUE, "Right Encoder"=w326, "Left Encoder"=w325) -> ("Right Encoder Out"=w329:T27, "Left Encoder Out"=w330:T27)  [unwired: 6 in, 1 out]
          n200 = while {
            shift-right: [w430] -> w311
            shift-left: w328 -> [w431]
            shift-right: [FALSE] -> _
            shift-left: TRUE -> [w416]
            shift-right: [w417] -> w313
            shift-left: w329 -> [w414]
            shift-right: [w418] -> w314
            shift-left: w330 -> [w415]
            shift-right: [w412] -> w312
            shift-left: w327 -> [w426]
            shift-right: [w406] -> w315
            shift-left: w324 -> [w407]
            tunnel: w310 -> [w401]
            stop <- w399 stop-if-true
            # "14.5 seconds"
            # "Elevator active - neutral\nresets to next shoot angle"
            # "Drive Forward (3)"
            n201 = disable-structure shown="Enabled" {
              disable-tunnel: w426 -> [w435 w439]
              disable-tunnel: w416 -> [w434 _]
              disable-tunnel: [w433 w439] -> w413
              frame Disabled {
                n202 = case shown="True" w434 {
                  tunnel: w435 -> [w436 w438]
                  tunnel: [w436 w437] -> w433
                  frame False {
                  }
                  frame True {
                    n203 = call <vilib>:"WPI_GyroReset.vi"("GyroDevRef"=w438) -> ("GyroDevRef"=w437:T21)  [unwired: 9 in, 1 out]
                  }
                }
              }
              frame Enabled {
              }
            }
            n204 = Wait (ms)(milliseconds to wait=u32 40) -> ()  [unwired: 1 out]
            n205 = local read "Auto Setpoints"() -> (w394:T3)
            n206 = Unbundle By Name(w394) -> ("Distance 3"=w419:dbl, "Two Disc Distance 3"=w409:dbl)
            n207 = call <vilib>:"WPI_GyroGetAngle.vi"("GyroDevRef"=w413) -> ("Angle"=w411:dbl, "GyroDevRef"=w412:T21)  [unwired: 7 in, 2 out]
            n208 = call "Read Encoders.vi"("Reset"=FALSE, "Right Encoder"=w414, "Left Encoder"=w415) -> ("Encoder Values"=w396:T31, "Right Encoder Out"=w417:T27, "Left Encoder Out"=w418:T27)  [unwired: 6 in]
            n209 = global read "Robot Global Data.vi" "UDP Packet"() -> (w398:T15)
            n210 = Unbundle By Name(w398) -> ("Auto Speed Constants"=w397:T19)
            n211 = Tick Count (ms)() -> (millisecond timer value=w405:u32)
            n212 = local read "Distance PID"() -> (w395:T1)
            n213 = Subtract(x=w405, y=w401) -> (x-y=w404:u32)
            n214 = Greater Or Equal?(x=w404, y=u32 14500) -> (x >= y?=w402:bool)
            n215 = call "AutoSpeed.vi"("Auto Speed Constants"=w397, "Encoder Values"=w396, "Two Disc Distance"=w409, "Reinitialize"=w416, "PID settings"=w395, "Target Distance"=w419) -> ("Finish"=w400:bool, "Backward"=w425:bool, "Y axis Speed"=w424:dbl, "Two Disc Loading"=w408:bool)  [unwired: 2 in]
            n216 = Bundle By Name(cluster=w407, "Load"=TRUE, "Shoot"=FALSE, "Elevator"=TRUE, "Two Discs"=w408) -> (w406:T6)
            n217 = Compound Arithmetic op=OR(w400, w402) -> (w399:bool)
            n218 = call "Auto Encoder Steering.vi"("Backward"=w425, "Gyro Angle"=w411) -> ("Steering"=w423:dbl)  [unwired: 8 in, 1 out]
            n219 = global write "Robot Global Data.vi" "Auton Commands"(w406) -> ()
            n220 = local write "Steering"(w423) -> ()
            n221 = local write "Y axis Speed"(w424) -> ()
            n222 = call-poly <vilib>:"WPI_RobotDriveArcadeDrive.vi"("Y axis value"=w424, "X axis value"=w423, "RobotDriveDevRef"=w431) -> ("Motor Values"=w429:dbl[], "RobotDriveDevRef"=w430:T7)  [unwired: 1 in, 6 out]
            n223 = call <vilib>:"SD Write Numeric Array.vi"("Numeric Array"=w429, "Name"="RobotDrive Motors") -> ()  [unwired: 8 in, 2 out]
          }
        }
        frame True {
          # "Spin - towards goal"
          # "Drive forward (3)"
          # "Spin - towards goal"
          # "Drive backwards (2) to center of field"
          # "Drive forward (1) and pickup discs"
          # "Arc backwards to the RIGHT"
          n224 = while {
            tunnel: w559 -> [w832]
            shift-right: [w826] -> w567
            shift-left: w608 -> [w828]
            shift-right: [w825] -> w566
            shift-left: w607 -> [w827]
            shift-right: [w813] -> w565
            shift-left: w606 -> [w814]
            shift-right: [w824] -> w564
            shift-left: w605 -> [w809]
            shift-right: [w823] -> w555
            shift-left: w609 -> [w840]
            shift-right: [FALSE ("Reset")] -> _
            shift-left: TRUE ("Reset") -> [w808]
            stop <- w831 stop-if-true
            # "14.5 seconds"
            n225 = global read "Robot Global Data.vi" "UDP Packet"() -> (w821:T15)
            n226 = Unbundle By Name(w821) -> ("Auto Speed Constants"=w820:T19)
            n227 = Wait (ms)(milliseconds to wait=u32 40) -> ()  [unwired: 1 out]
            n228 = local read "Auto-Center Line"() -> (w822:T2)
            n229 = Unbundle By Name(w822) -> ("Arc Turn Distance"=w818:dbl)
            n230 = local read "Distance PID"() -> (w805:T1)
            n231 = call "Read Encoders.vi"("Reset"=FALSE, "Right Encoder"=w827, "Left Encoder"=w828) -> ("Encoder Values"=w806:T31, "Right Encoder Out"=w825:T27, "Left Encoder Out"=w826:T27)  [unwired: 6 in]
            n232 = Tick Count (ms)() -> (millisecond timer value=w833:u32)
            n233 = Bundle By Name(cluster=w840, "Load"=FALSE, "Shoot"=FALSE, "Elevator"=TRUE, "Two Discs"=FALSE) -> (w823:T6)
            n234 = call "AutoSpeed.vi"("Auto Speed Constants"=w820, "Encoder Values"=w806, "Two Disc Distance"=0.0, "Reinitialize"=w808, "PID settings"=w805, "Target Distance"=w818) -> ("Finish"=w816:bool, "Backward"=w815:bool, "Y axis Speed"=w817:dbl)  [unwired: 2 in, 1 out]
            n235 = call <vilib>:"WPI_GyroGetAngle.vi"("GyroDevRef"=w814) -> ("Angle"=w812:dbl, "GyroDevRef"=w813:T21)  [unwired: 7 in, 2 out]
            n236 = Subtract(x=w833, y=w832) -> (x-y=w834:u32)
            n237 = Greater Or Equal?(x=w834, y=u32 14500) -> (x >= y?=w830:bool)
            n238 = call "Auto Encoder Steering.vi"("Backward"=w815, "Gyro Angle"=w812, "Angle setpoint"=0.0) -> ("Steering"=w810:dbl)  [unwired: 7 in, 1 out]
            n239 = global write "Robot Global Data.vi" "Auton Commands"(w823) -> ()
            n240 = call-poly <vilib>:"WPI_RobotDriveArcadeDrive.vi"("Y axis value"=w817, "X axis value"=w810, "RobotDriveDevRef"=w809) -> ("RobotDriveDevRef"=w824:T7)  [unwired: 1 in, 7 out]
            n241 = Compound Arithmetic op=OR(w816, w830) -> (w831:bool)
          }
          n242 = Unbundle By Name(w555) -> ("Low Gear"=w554:bool)
          n243 = call "Read Encoders.vi"("Reset"=TRUE, "Right Encoder"=w566, "Left Encoder"=w567) -> ("Right Encoder Out"=w570:T27, "Left Encoder Out"=w569:T27)  [unwired: 6 in, 1 out]
          n244 = while {
            shift-right: [w646] -> w563
            shift-left: w564 -> [w647]
            shift-right: [w627] -> w560
            shift-left: w569 -> [w629]
            shift-right: [w626] -> w561
            shift-left: w570 -> [w628]
            shift-right: [w648] -> w562
            shift-left: w565 -> [w649]
            shift-right: [w641] -> w556
            shift-left: w555 -> [w642]
            tunnel: w559 -> [w611]
            stop <- w635 stop-if-true
            # "force Low Gear"
            # "Wait for: spin angle\nOR encoder distance"
            # "14.5 seconds"
            n245 = global read "Robot Global Data.vi" "UDP Packet"() -> (w614:T15)
            n246 = Unbundle By Name(w614) -> ("Spin PID gains"=w613:T20, "Spin output range"=w612:cluster{"output high":dbl, "output low":dbl})
            n247 = local read "Auto-Center Line"() -> (w619:T2)
            n248 = Unbundle By Name(w619) -> ("Spin Distance"=w616:dbl, "Spin Angle"=w618:dbl, "Spin Angle tolerance"=w617:dbl, "Spin y-axis"=w615:dbl)
            n249 = call <vilib>:"WPI_GyroGetAngle.vi"("GyroDevRef"=w649) -> ("Angle"=w632:dbl, "GyroDevRef"=w648:T21)  [unwired: 7 in, 2 out]
            n250 = Bundle By Name(cluster=w642, "Load"=FALSE, "Shoot"=FALSE, "Elevator"=TRUE, "Two Discs"=FALSE, "Low Gear"=TRUE) -> (w641:T6)
            n251 = global write "Robot Global Data.vi" "Auton Commands"(w641) -> ()
            n252 = call "Read Encoders.vi"("Right Encoder"=w628, "Left Encoder"=w629) -> ("Encoder Values"=w625:T31, "Right Encoder Out"=w626:T27, "Left Encoder Out"=w627:T27)  [unwired: 7 in]
            n253 = Unbundle By Name(w625) -> ("Avg Distance"=w620:dbl)
            n254 = Subtract(x=w632, y=w618) -> (x-y=w633:dbl)
            n255 = call-poly <vilib>:"PID.vi"("output range"=w612, "PID gains"=w613, "process variable"=w632, "setpoint"=w618) -> ("output"=w631:dbl)  [unwired: 6 in, 1 out]
            n256 = Tick Count (ms)() -> (millisecond timer value=w638:u32)
            n257 = Absolute Value(x=w633) -> (abs(x)=w634:dbl)
            n258 = Less Or Equal?(x=w634, y=w617) -> (x <= y?=w624:bool)
            n259 = Subtract(x=w638, y=w611) -> (x-y=w637:u32)
            n260 = Wait (ms)(milliseconds to wait=u32 40) -> ()  [unwired: 1 out]
            n261 = Greater Or Equal?(x=w637, y=u32 14500) -> (x >= y?=w639:bool)
            n262 = Greater Or Equal?(x=w620, y=w616) -> (x >= y?=w621:bool)
            n263 = Not Equal To 0?(x=w615) -> (x != 0?=w622:bool)
            n264 = call-poly <vilib>:"WPI_RobotDriveArcadeDrive.vi"("Y axis value"=w615, "X axis value"=w631, "RobotDriveDevRef"=w647) -> ("RobotDriveDevRef"=w646:T7)  [unwired: 1 in, 7 out]
            n265 = Select(t=w621, s=w622, f=w624) -> (s? t:f=w623:bool)
            n266 = Compound Arithmetic op=OR(w623, w639) -> (w635:bool)
          }
          n267 = Bundle By Name(cluster=w556, "Low Gear"=w554) -> (w557:T6)
          n268 = call <vilib>:"WPI_GyroReset.vi"("GyroDevRef"=w562) -> ("GyroDevRef"=w601:T21)  [unwired: 9 in, 1 out]
          n269 = call "Read Encoders.vi"("Reset"=TRUE, "Right Encoder"=w561, "Left Encoder"=w560) -> ("Right Encoder Out"=w603:T27, "Left Encoder Out"=w604:T27)  [unwired: 6 in, 1 out]
          n270 = while {
            shift-right: [w800] -> w599
            shift-left: w557 -> [w801]
            shift-right: [w796] -> w596
            shift-left: w603 -> [w798]
            shift-right: [w797] -> w597
            shift-left: w604 -> [w799]
            shift-right: [w793] -> w571
            shift-left: w601 -> [w794]
            tunnel: w559 -> [w789]
            shift-right: [w785] -> w593
            shift-left: w563 -> [w771]
            shift-right: [FALSE ("Reset")] -> _
            shift-left: TRUE ("Reset") -> [w780]
            stop <- w787 stop-if-true
            # "14.5 seconds"
            n271 = local read "Auto-Center Line"() -> (w774:T2)
            n272 = Unbundle By Name(w774) -> ("Distance 1"=w773:dbl, "Two Disc Distance 1"=w772:dbl)
            n273 = call <vilib>:"WPI_GyroGetAngle.vi"("GyroDevRef"=w794) -> ("Angle"=w784:dbl, "GyroDevRef"=w793:T21)  [unwired: 7 in, 2 out]
            n274 = call "Read Encoders.vi"("Reset"=FALSE, "Right Encoder"=w798, "Left Encoder"=w799) -> ("Encoder Values"=w770:T31, "Right Encoder Out"=w796:T27, "Left Encoder Out"=w797:T27)  [unwired: 6 in]
            n275 = Wait (ms)(milliseconds to wait=u32 40) -> ()  [unwired: 1 out]
            n276 = global read "Robot Global Data.vi" "UDP Packet"() -> (w776:T15)
            n277 = Unbundle By Name(w776) -> ("Auto Speed Constants"=w775:T19)
            n278 = local read "Distance PID"() -> (w769:T1)
            n279 = Tick Count (ms)() -> (millisecond timer value=w790:u32)
            n280 = Subtract(x=w790, y=w789) -> (x-y=w791:u32)
            n281 = Greater Or Equal?(x=w791, y=u32 14500) -> (x >= y?=w788:bool)
            n282 = call "AutoSpeed.vi"("Auto Speed Constants"=w775, "Encoder Values"=w770, "Two Disc Distance"=w772, "Reinitialize"=w780, "PID settings"=w769, "Target Distance"=w773) -> ("Finish"=w781:bool, "Backward"=w782:bool, "Y axis Speed"=w777:dbl, "Two Disc Loading"=w778:bool)  [unwired: 2 in]
            n283 = Compound Arithmetic op=OR(w781, w788) -> (w787:bool)
            n284 = call "Auto Encoder Steering.vi"("Backward"=w782, "Gyro Angle"=w784) -> ("Steering"=w783:dbl)  [unwired: 8 in, 1 out]
            n285 = Bundle By Name(cluster=w801, "Load"=TRUE, "Shoot"=FALSE, "Elevator"=TRUE, "Two Discs"=w778) -> (w800:T6)
            n286 = global write "Robot Global Data.vi" "Auton Commands"(w800) -> ()
            n287 = call-poly <vilib>:"WPI_RobotDriveArcadeDrive.vi"("Y axis value"=w777, "X axis value"=w783, "RobotDriveDevRef"=w771) -> ("RobotDriveDevRef"=w785:T7)  [unwired: 1 in, 7 out]
          }
          n288 = call "Read Encoders.vi"("Reset"=TRUE, "Right Encoder"=w596, "Left Encoder"=w597) -> ("Right Encoder Out"=w594:T27, "Left Encoder Out"=w595:T27)  [unwired: 6 in, 1 out]
          n289 = while {
            shift-right: [w764] -> w553
            shift-left: w599 -> [w763]
            shift-right: [w759] -> w591
            shift-left: w595 -> [w761]
            shift-right: [w758] -> w589
            shift-left: w594 -> [w760]
            shift-right: [w751] -> w578
            shift-left: w571 -> [w752]
            tunnel: w559 -> [w739]
            shift-right: [w750] -> w587
            shift-left: w593 -> [w737]
            shift-right: [FALSE ("Reset")] -> _
            shift-left: TRUE ("Reset") -> [w742]
            stop <- w753 stop-if-true
            # "force Low Gear"
            # "14.5 seconds"
            n290 = global read "Robot Global Data.vi" "UDP Packet"() -> (w748:T15)
            n291 = Unbundle By Name(w748) -> ("Auto Speed Constants"=w749:T19)
            n292 = local read "Auto-Center Line"() -> (w738:T2)
            n293 = Unbundle By Name(w738) -> ("Distance 2"=w735:dbl, "Two Disc Distance 2"=w736:dbl)
            n294 = call "Read Encoders.vi"("Reset"=FALSE, "Right Encoder"=w760, "Left Encoder"=w761) -> ("Encoder Values"=w734:T31, "Right Encoder Out"=w758:T27, "Left Encoder Out"=w759:T27)  [unwired: 6 in]
            n295 = Wait (ms)(milliseconds to wait=u32 40) -> ()  [unwired: 1 out]
            n296 = call <vilib>:"WPI_GyroGetAngle.vi"("GyroDevRef"=w752) -> ("Angle"=w744:dbl, "GyroDevRef"=w751:T21)  [unwired: 7 in, 2 out]
            n297 = local read "Distance PID"() -> (w733:T1)
            n298 = Tick Count (ms)() -> (millisecond timer value=w756:u32)
            n299 = Subtract(x=w756, y=w739) -> (x-y=w755:u32)
            n300 = call "AutoSpeed.vi"("Auto Speed Constants"=w749, "Encoder Values"=w734, "Two Disc Distance"=w736, "Reinitialize"=w742, "PID settings"=w733, "Target Distance"=w735) -> ("Finish"=w740:bool, "Backward"=w747:bool, "Y axis Speed"=w746:dbl, "Two Disc Loading"=w743:bool)  [unwired: 2 in]
            n301 = Greater Or Equal?(x=w755, y=u32 14500) -> (x >= y?=w757:bool)
            n302 = call "Auto Encoder Steering.vi"("Backward"=w747, "Gyro Angle"=w744) -> ("Steering"=w745:dbl)  [unwired: 8 in, 1 out]
            n303 = Compound Arithmetic op=OR(w740, w757) -> (w753:bool)
            n304 = Bundle By Name(cluster=w763, "Load"=TRUE, "Shoot"=FALSE, "Elevator"=TRUE, "Two Discs"=w743) -> (w764:T6)
            n305 = global write "Robot Global Data.vi" "Auton Commands"(w764) -> ()
            n306 = call-poly <vilib>:"WPI_RobotDriveArcadeDrive.vi"("Y axis value"=w746, "X axis value"=w745, "RobotDriveDevRef"=w737) -> ("RobotDriveDevRef"=w750:T7)  [unwired: 1 in, 7 out]
          }
          n307 = Unbundle By Name(w553) -> ("Low Gear"=w550:bool)
          n308 = call "Read Encoders.vi"("Reset"=TRUE, "Right Encoder"=w589, "Left Encoder"=w591) -> ("Right Encoder Out"=w581:T27, "Left Encoder Out"=w582:T27)  [unwired: 6 in, 1 out]
          n309 = while {
            shift-right: [w686] -> w586
            shift-left: w587 -> [w687]
            shift-right: [w666] -> w580
            shift-left: w582 -> [w668]
            shift-right: [w665] -> w579
            shift-left: w581 -> [w667]
            shift-right: [w688] -> w577
            shift-left: w578 -> [w689]
            shift-right: [w681] -> w552
            shift-left: w553 -> [w682]
            tunnel: w559 -> [w675]
            stop <- w674 stop-if-true
            # "force Low Gear"
            # "Wait for: spin angle\nOR encoder distance"
            # "14.5 seconds"
            n310 = global read "Robot Global Data.vi" "UDP Packet"() -> (w653:T15)
            n311 = Unbundle By Name(w653) -> ("Spin PID gains"=w652:T20, "Spin output range"=w651:cluster{"output high":dbl, "output low":dbl})
            n312 = local read "Auto-Center Line"() -> (w658:T2)
            n313 = Unbundle By Name(w658) -> ("Spin Distance 2"=w655:dbl, "Spin Angle 2"=w657:dbl, "Spin Angle tolerance 2"=w656:dbl, "Spin y-axis 2"=w654:dbl)
            n314 = call <vilib>:"WPI_GyroGetAngle.vi"("GyroDevRef"=w689) -> ("Angle"=w671:dbl, "GyroDevRef"=w688:T21)  [unwired: 7 in, 2 out]
            n315 = Bundle By Name(cluster=w682, "Load"=FALSE, "Shoot"=FALSE, "Elevator"=TRUE, "Two Discs"=FALSE, "Low Gear"=TRUE) -> (w681:T6)
            n316 = global write "Robot Global Data.vi" "Auton Commands"(w681) -> ()
            n317 = call "Read Encoders.vi"("Right Encoder"=w667, "Left Encoder"=w668) -> ("Encoder Values"=w664:T31, "Right Encoder Out"=w665:T27, "Left Encoder Out"=w666:T27)  [unwired: 7 in]
            n318 = Unbundle By Name(w664) -> ("Avg Distance"=w659:dbl)
            n319 = Subtract(x=w671, y=w657) -> (x-y=w672:dbl)
            n320 = call-poly <vilib>:"PID.vi"("output range"=w651, "PID gains"=w652, "process variable"=w671, "setpoint"=w657) -> ("output"=w670:dbl)  [unwired: 6 in, 1 out]
            n321 = Tick Count (ms)() -> (millisecond timer value=w678:u32)
            n322 = Absolute Value(x=w672) -> (abs(x)=w673:dbl)
            n323 = Less Or Equal?(x=w673, y=w656) -> (x <= y?=w663:bool)
            n324 = Subtract(x=w678, y=w675) -> (x-y=w677:u32)
            n325 = Wait (ms)(milliseconds to wait=u32 40) -> ()  [unwired: 1 out]
            n326 = Greater Or Equal?(x=w677, y=u32 14500) -> (x >= y?=w679:bool)
            n327 = Greater Or Equal?(x=w659, y=w655) -> (x >= y?=w660:bool)
            n328 = Not Equal To 0?(x=w654) -> (x != 0?=w661:bool)
            n329 = call-poly <vilib>:"WPI_RobotDriveArcadeDrive.vi"("Y axis value"=w654, "X axis value"=w670, "RobotDriveDevRef"=w687) -> ("RobotDriveDevRef"=w686:T7)  [unwired: 1 in, 7 out]
            n330 = Select(t=w660, s=w661, f=w663) -> (s? t:f=w662:bool)
            n331 = Compound Arithmetic op=OR(w662, w679) -> (w674:bool)
          }
          n332 = Bundle By Name(cluster=w552, "Low Gear"=w550) -> (w551:T6)
          n333 = call "Read Encoders.vi"("Reset"=TRUE, "Right Encoder"=w579, "Left Encoder"=w580) -> ("Right Encoder Out"=w583:T27, "Left Encoder Out"=w584:T27)  [unwired: 6 in, 1 out]
          n334 = while {
            shift-right: [w723] -> w576
            shift-left: w551 -> [w724]
            shift-right: [w718] -> w574
            shift-left: w583 -> [w720]
            shift-right: [w719] -> w575
            shift-left: w584 -> [w721]
            tunnel: w559 -> [w713]
            shift-right: [w711] -> w572
            shift-left: w586 -> [w695]
            shift-right: [FALSE ("Reset")] -> _
            shift-left: TRUE ("Reset") -> [w708]
            shift-right: [w704] -> w573
            shift-left: w577 -> [w705]
            stop <- w712 stop-if-true
            # "14.5 seconds"
            n335 = local read "Auto-Center Line"() -> (w699:T2)
            n336 = Unbundle By Name(w699) -> ("Spin Angle 2"=w698:dbl, "Distance 3"=w697:dbl, "Two Disc Distance 3"=w696:dbl)
            n337 = Wait (ms)(milliseconds to wait=u32 40) -> ()  [unwired: 1 out]
            n338 = call "Read Encoders.vi"("Reset"=FALSE, "Right Encoder"=w720, "Left Encoder"=w721) -> ("Encoder Values"=w691:T31, "Right Encoder Out"=w718:T27, "Left Encoder Out"=w719:T27)  [unwired: 6 in]
            n339 = call <vilib>:"WPI_GyroGetAngle.vi"("GyroDevRef"=w705) -> ("Angle"=w703:dbl, "GyroDevRef"=w704:T21)  [unwired: 7 in, 2 out]
            n340 = global read "Robot Global Data.vi" "UDP Packet"() -> (w710:T15)
            n341 = Unbundle By Name(w710) -> ("Auto Speed Constants"=w709:T19)
            n342 = local read "Distance PID"() -> (w690:T1)
            n343 = disable-structure shown="Enabled" {
              disable-tunnel: [w730 FALSE] -> w693
              disable-tunnel: _ -> [w729 _]
              frame Disabled {
                n344 = Absolute Value(x=w729) -> (abs(x)=w728:dbl)
                n345 = Less Or Equal?(x=w728, y=2.0) -> (x <= y?=w730:bool)
              }
              frame Enabled {
              }
            }
            n346 = Tick Count (ms)() -> (millisecond timer value=w715:u32)
            n347 = Subtract(x=w715, y=w713) -> (x-y=w716:u32)
            n348 = Greater Or Equal?(x=w716, y=u32 14500) -> (x >= y?=w714:bool)
            n349 = call "AutoSpeed.vi"("Auto Speed Constants"=w709, "Encoder Values"=w691, "Two Disc Distance"=w696, "Reinitialize"=w708, "PID settings"=w690, "Target Distance"=w697) -> ("Finish"=w700:bool, "Backward"=w702:bool, "Y axis Speed"=w707:dbl)  [unwired: 2 in, 1 out]
            n350 = Bundle By Name(cluster=w724, "Load"=w693, "Shoot"=FALSE, "Elevator"=TRUE, "Two Discs"=FALSE, "Warmup"=TRUE) -> (w723:T6)
            n351 = global write "Robot Global Data.vi" "Auton Commands"(w723) -> ()
            n352 = call "Auto Encoder Steering.vi"("Backward"=w702, "Gyro Angle"=w703, "Angle setpoint"=w698) -> ("Steering"=w701:dbl)  [unwired: 7 in, 1 out]
            n353 = Compound Arithmetic op=OR(w700, w714) -> (w712:bool)
            n354 = call-poly <vilib>:"WPI_RobotDriveArcadeDrive.vi"("Y axis value"=w707, "X axis value"=w701, "RobotDriveDevRef"=w695) -> ("RobotDriveDevRef"=w711:T7)  [unwired: 1 in, 7 out]
          }
        }
      }
      n355 = while {
        shift-right: [w213] -> w153
        shift-left: w152 -> [w214]
        shift-right: [FALSE] -> _
        shift-left: TRUE -> [w209]
        shift-right: [w206] -> _
        shift-left: _ -> [w207]
        stop <- w202 stop-if-true
        n356 = Wait (ms)(milliseconds to wait=u32 40) -> ()  [unwired: 1 out]
        n357 = case shown="False" w209 {
          tunnel: [w215 w216] -> w206
          tunnel: w207 -> [w215 _]
          frame False {
          }
          frame True {
            n358 = Tick Count (ms)() -> (millisecond timer value=w216:u32)
          }
        }
        n359 = global read "Robot Global Data.vi" "UDP Packet"() -> (w211:T15)
        n360 = Unbundle By Name(w211) -> ("Auto Stop Throttle"=w210:dbl, "Auto Stop Duration"=w203:dbl)
        n361 = Tick Count (ms)() -> (millisecond timer value=w205:u32)
        n362 = call-poly <vilib>:"WPI_RobotDriveArcadeDrive.vi"("Y axis value"=w210, "X axis value"=0.0, "RobotDriveDevRef"=w214) -> ("RobotDriveDevRef"=w213:T7)  [unwired: 1 in, 7 out]
        n363 = Subtract(x=w205, y=w206) -> (x-y=w204:u32)
        n364 = Greater Or Equal?(x=w204, y=w203) -> (x >= y?=w202:bool)
      }
      n365 = while {
        shift-right: [w265] -> w159
        shift-left: w153 -> [w265]
        stop <- TRUE stop-if-true
        # "Even if IR's didn't read\ndiscs, fire X discs"
        n366 = disable-structure shown="Enabled" {
          disable-tunnel: [w268 w269] -> w264
          frame Disabled {
            n367 = call <vilib>:"SD Read Number.vi"("Name"="Auto/Disc Count 3") -> ("Numeric"=w268:dbl)  [unwired: 8 in, 2 out]
          }
          frame Enabled {
            n368 = local read "Auto Setpoints"() -> (w270:T3)
            n369 = Unbundle By Name(w270) -> ("Disc Count 3"=w269:dbl)
          }
        }
        n370 = disable-structure shown="Enabled" {
          disable-tunnel: [w272 w274] -> _
          disable-tunnel: w264 -> [w271 w274]
          frame Disabled {
            n371 = global read "Robot Global Data.vi" "Disc Count"() -> (w273:dbl)
            n372 = Max & Min(x=w271, y=w273) -> (max(x,y)=w272:dbl)  [unwired: 1 out]
          }
          frame Enabled {
          }
        }
        n373 = global write "Robot Global Data.vi" "Disc Count"(w264) -> ()
      }
      n374 = while {
        shift-right: [w303] -> w165
        shift-left: w159 -> [w304]
        shift-right: [w286] -> w166
        shift-left: w158 -> [w293]
        tunnel: TRUE -> [w290]
        shift-right: [w289] -> _
        shift-left: _ -> [w288]
        tunnel: w155 -> [w278]
        stop <- w275 stop-if-true
        (unwired) FALSE
        w301 = 0.0 ("Y axis value")
        # "14.5 seconds"
        # "Shoot (3)"
        n375 = local read "Auto Setpoints"() -> (w285:T3)
        n376 = Unbundle By Name(w285) -> ("Shoot Angle 3"=w284:dbl, "Shoot Time 3"=w283:dbl)
        n377 = Tick Count (ms)() -> (millisecond timer value=w287:u32)
        n378 = case shown="True" w290 {
          tunnel: [w308 w309] -> w289
          tunnel: w288 -> [w308 _]
          tunnel: w287 -> [_ w309]
          frame False {
          }
          frame True {
          }
        }
        n379 = disable-structure shown="Enabled" {
          disable-tunnel: [w305 w307] -> w291
          disable-tunnel: w283 -> [_ w307]
          frame Disabled {
            n380 = call <vilib>:"SD Read Number.vi"("Name"="Auto/Shoot Time 3") -> ("Numeric"=w305:dbl)  [unwired: 8 in, 2 out]
          }
          frame Enabled {
          }
        }
        n381 = Wait (ms)(milliseconds to wait=u32 40) -> ()  [unwired: 1 out]
        n382 = Tick Count (ms)() -> (millisecond timer value=w282:u32)
        n383 = global read "Robot Global Data.vi" "Disc Count"() -> (w299:dbl)
        n384 = Bundle By Name(cluster=w293, "Load"=FALSE, "Shoot"=TRUE, "Azimuth"=TRUE, "Elevator"=TRUE, "Shoot Angle"=w284, "Neutral Angle"=w284) -> (w286:T6)
        n385 = call-poly <vilib>:"WPI_RobotDriveArcadeDrive.vi"("Y axis value"=w301, "X axis value"=w301, "RobotDriveDevRef"=w304) -> ("Motor Values"=w302:dbl[], "RobotDriveDevRef"=w303:T7)  [unwired: 1 in, 6 out]
        n386 = global write "Robot Global Data.vi" "Auton Commands"(w286) -> ()
        n387 = Subtract(x=w282, y=w278) -> (x-y=w281:u32)
        n388 = Subtract(x=w287, y=w289) -> (x-y=w292:u32)
        n389 = call <vilib>:"SD Write Numeric Array.vi"("Numeric Array"=w302, "Name"="RobotDrive Motors") -> ()  [unwired: 8 in, 2 out]
        n390 = Greater Or Equal?(x=w281, y=u32 14500) -> (x >= y?=w279:bool)
        n391 = Greater Or Equal?(x=w292, y=w291) -> (x >= y?=w277:bool)
        n392 = Less Or Equal To 0?(x=w299) -> (x <= 0?=w276:bool)
        n393 = Compound Arithmetic op=OR(w276, w277, w279) -> (w275:bool)
      }
      n394 = call "Read Encoders.vi"("Reset"=TRUE, "Right Encoder"=w157, "Left Encoder"=w151) -> ("Right Encoder Out"=w161:T27, "Left Encoder Out"=w162:T27)  [unwired: 6 in, 1 out]
      n395 = while {
        shift-right: [w254] -> w149
        shift-left: w165 -> [w255]
        shift-right: [FALSE] -> _
        shift-left: TRUE -> [w240]
        shift-right: [w241] -> _
        shift-left: w161 -> [w238]
        shift-right: [w242] -> _
        shift-left: w162 -> [w239]
        shift-right: [w236] -> _
        shift-left: w156 -> [w250]
        shift-right: [w230] -> w150
        shift-left: w166 -> [w231]
        tunnel: w155 -> [w225]
        stop <- w223 stop-if-true
        # "14.5 seconds"
        # "[if distance is negative]"
        # "Elevator active - neutral\nresets to next shoot angle"
        # "Drive Backward (4)"
        n396 = disable-structure shown="Enabled" {
          disable-tunnel: w250 -> [w259 w263]
          disable-tunnel: w240 -> [w258 _]
          disable-tunnel: [w257 w263] -> w237
          frame Disabled {
            n397 = case shown="True" w258 {
              tunnel: w259 -> [w260 w262]
              tunnel: [w260 w261] -> w257
              frame False {
              }
              frame True {
                n398 = call <vilib>:"WPI_GyroReset.vi"("GyroDevRef"=w262) -> ("GyroDevRef"=w261:T21)  [unwired: 9 in, 1 out]
              }
            }
          }
          frame Enabled {
          }
        }
        n399 = Wait (ms)(milliseconds to wait=u32 40) -> ()  [unwired: 1 out]
        n400 = local read "Auto Setpoints"() -> (w218:T3)
        n401 = Unbundle By Name(w218) -> ("Distance 4"=w243:dbl, "Two Disc Distance 4"=w233:dbl)
        n402 = call <vilib>:"WPI_GyroGetAngle.vi"("GyroDevRef"=w237) -> ("Angle"=w235:dbl, "GyroDevRef"=w236:T21)  [unwired: 7 in, 2 out]
        n403 = call "Read Encoders.vi"("Reset"=FALSE, "Right Encoder"=w238, "Left Encoder"=w239) -> ("Encoder Values"=w219:T31, "Right Encoder Out"=w241:T27, "Left Encoder Out"=w242:T27)  [unwired: 6 in]
        n404 = local read "Distance PID"() -> (w217:T1)
        n405 = global read "Robot Global Data.vi" "UDP Packet"() -> (w222:T15)
        n406 = Unbundle By Name(w222) -> ("Auto Speed Constants"=w221:T19)
        n407 = Tick Count (ms)() -> (millisecond timer value=w229:u32)
        n408 = Subtract(x=w229, y=w225) -> (x-y=w228:u32)
        n409 = Greater Or Equal?(x=w228, y=u32 14500) -> (x >= y?=w226:bool)
        n410 = call "AutoSpeed.vi"("Auto Speed Constants"=w221, "Encoder Values"=w219, "Two Disc Distance"=w233, "Reinitialize"=w240, "PID settings"=w217, "Target Distance"=w243) -> ("Finish"=w224:bool, "Backward"=w249:bool, "Y axis Speed"=w248:dbl, "Two Disc Loading"=w232:bool)  [unwired: 2 in]
        n411 = Compound Arithmetic op=OR(w224, w226) -> (w223:bool)
        n412 = Bundle By Name(cluster=w231, "Load"=TRUE, "Shoot"=FALSE, "Elevator"=TRUE, "Two Discs"=w232, "Warmup"=FALSE) -> (w230:T6)
        n413 = call "Auto Encoder Steering.vi"("Backward"=w249, "Gyro Angle"=w235) -> ("Steering"=w247:dbl)  [unwired: 8 in, 1 out]
        n414 = global write "Robot Global Data.vi" "Auton Commands"(w230) -> ()
        n415 = local write "Steering"(w247) -> ()
        n416 = local write "Y axis Speed"(w248) -> ()
        n417 = call-poly <vilib>:"WPI_RobotDriveArcadeDrive.vi"("Y axis value"=w248, "X axis value"=w247, "RobotDriveDevRef"=w255) -> ("Motor Values"=w253:dbl[], "RobotDriveDevRef"=w254:T7)  [unwired: 1 in, 6 out]
        n418 = call <vilib>:"SD Write Numeric Array.vi"("Numeric Array"=w253, "Name"="RobotDrive Motors") -> ()  [unwired: 8 in, 2 out]
      }
    }
    frame True {
      n419 = call <vilib>:"WPI_EncoderRefNum Registry Get.vi"("refnum name"="Drive Encoder Left") -> ("EncoderDevRef"=w902:T27)  [unwired: 9 in, 1 out]
      n420 = call <vilib>:"WPI_EncoderRefNum Registry Get.vi"("refnum name"="Drive Encoder Right") -> ("EncoderDevRef"=w901:T27)  [unwired: 9 in, 1 out]
      n421 = call "Read Encoders.vi"("Reset"=TRUE, "Right Encoder"=w901, "Left Encoder"=w902) -> ("Right Encoder Out"=w899:T27, "Left Encoder Out"=w900:T27)  [unwired: 6 in, 1 out]
      n422 = while {
        shift-right: [FALSE ("Reset")] -> _
        shift-left: TRUE ("Reset") -> [w985]
        shift-right: [w982] -> w890
        shift-left: w906 -> [w983]
        shift-right: [w979] -> w886
        shift-left: w900 -> [w981]
        shift-right: [w978] -> w885
        shift-left: w899 -> [w980]
        shift-right: [w975] -> w891
        shift-left: w897 -> [w976]
        tunnel: w887 -> [w974]
        shift-right: [w973] -> w894
        shift-left: w898 -> [w977]
        stop <- w986 stop-if-true
        # "14.5 seconds"
        n423 = global read "Robot Global Data.vi" "UDP Packet"() -> (w995:T15)
        n424 = Unbundle By Name(w995) -> ("Auto Speed Constants"=w994:T19)
        n425 = local read "Distance PID"() -> (w968:T1)
        n426 = local read "Auto Setpoints"() -> (w971:T3)
        n427 = Wait (ms)(milliseconds to wait=u32 40) -> ()  [unwired: 1 out]
        n428 = Unbundle By Name(w971) -> ("Distance 1"=w970:dbl)
        n429 = call "Read Encoders.vi"("Reset"=FALSE, "Right Encoder"=w980, "Left Encoder"=w981) -> ("Encoder Values"=w969:T31, "Right Encoder Out"=w978:T27, "Left Encoder Out"=w979:T27)  [unwired: 6 in]
        n430 = Tick Count (ms)() -> (millisecond timer value=w998:u32)
        n431 = Bundle By Name(cluster=w977, "Load"=FALSE, "Shoot"=FALSE, "Elevator"=TRUE, "Two Discs"=FALSE) -> (w973:T6)
        n432 = call "AutoSpeed.vi"("Auto Speed Constants"=w994, "Encoder Values"=w969, "Two Disc Distance"=0.0, "Reinitialize"=w985, "PID settings"=w968, "Target Distance"=w970) -> ("Finish"=w991:bool, "Backward"=w990:bool, "Y axis Speed"=w992:dbl)  [unwired: 2 in, 1 out]
        n433 = call <vilib>:"WPI_GyroGetAngle.vi"("GyroDevRef"=w976) -> ("Angle"=w989:dbl, "GyroDevRef"=w975:T21)  [unwired: 7 in, 2 out]
        n434 = Subtract(x=w998, y=w974) -> (x-y=w999:u32)
        n435 = Greater Or Equal?(x=w999, y=u32 14500) -> (x >= y?=w997:bool)
        n436 = call "Auto Encoder Steering.vi"("Backward"=w990, "Gyro Angle"=w989, "Angle setpoint"=0.0) -> ("Steering"=w987:dbl)  [unwired: 7 in, 1 out]
        n437 = global write "Robot Global Data.vi" "Auton Commands"(w973) -> ()
        n438 = call-poly <vilib>:"WPI_RobotDriveArcadeDrive.vi"("Y axis value"=w992, "X axis value"=w987, "RobotDriveDevRef"=w983) -> ("RobotDriveDevRef"=w982:T7)  [unwired: 1 in, 7 out]
        n439 = Compound Arithmetic op=OR(w991, w997) -> (w986:bool)
      }
      n440 = call "Read Encoders.vi"("Reset"=TRUE, "Right Encoder"=w885, "Left Encoder"=w886) -> ("Right Encoder Out"=w883:T27, "Left Encoder Out"=w884:T27)  [unwired: 6 in, 1 out]
      n441 = while {
        shift-right: [w928] -> w882
        shift-left: w884 -> [w928]
        shift-right: [w927] -> w881
        shift-left: w883 -> [w927]
        shift-right: [w926] -> w889
        shift-left: w891 -> [w926]
        shift-right: [w924] -> w888
        shift-left: w890 -> [w925]
        tunnel: w887 -> [w919]
        shift-right: [FALSE ("Reset")] -> _
        shift-left: TRUE ("Reset") -> [w913]
        shift-right: [w912] -> _
        shift-left: _ -> [w911]
        stop <- w918 stop-if-true
        w923 = 0.0 ("X axis value")
        # "14.5 seconds"
        n442 = Tick Count (ms)() -> (millisecond timer value=w910:u32)
        n443 = Subtract(x=w910, y=w919) -> (x-y=w921:u32)
        n444 = case shown="False" w913 {
          tunnel: [w929 w930] -> w912
          tunnel: w910 -> [_ w930]
          tunnel: w911 -> [w929 _]
          frame False {
          }
          frame True {
          }
        }
        n445 = Greater Or Equal?(x=w921, y=u32 14500) -> (x >= y?=w922:bool)
        n446 = Wait (ms)(milliseconds to wait=u32 40) -> ()  [unwired: 1 out]
        n447 = local read "Auto Setpoints"() -> (w917:T3)
        n448 = Unbundle By Name(w917) -> ("Shoot Time 1"=w909:dbl)
        n449 = Subtract(x=w910, y=w912) -> (x-y=w914:u32)
        n450 = Greater Or Equal?(x=w914, y=w909) -> (x >= y?=w908:bool)
        n451 = Compound Arithmetic op=OR(w908, w922) -> (w918:bool)
        n452 = call-poly <vilib>:"WPI_RobotDriveArcadeDrive.vi"("Y axis value"=w923, "X axis value"=w923, "RobotDriveDevRef"=w925) -> ("RobotDriveDevRef"=w924:T7)  [unwired: 1 in, 7 out]
      }
      n453 = while {
        shift-right: [FALSE ("Reset")] -> _
        shift-left: TRUE ("Reset") -> [w948]
        shift-right: [w945] -> w893
        shift-left: w888 -> [w946]
        shift-right: [w942] -> _
        shift-left: w882 -> [w944]
        shift-right: [w941] -> _
        shift-left: w881 -> [w943]
        shift-right: [w938] -> _
        shift-left: w889 -> [w939]
        shift-right: [w937] -> w892
        shift-left: w894 -> [w940]
        tunnel: w887 -> [w933]
        stop <- w949 stop-if-true
        # "14.5 seconds"
        n454 = global read "Robot Global Data.vi" "UDP Packet"() -> (w958:T15)
        n455 = Unbundle By Name(w958) -> ("Auto Speed Constants"=w957:T19)
        n456 = local read "Auto Setpoints"() -> (w935:T3)
        n457 = local read "Distance PID"() -> (w931:T1)
        n458 = Wait (ms)(milliseconds to wait=u32 40) -> ()  [unwired: 1 out]
        n459 = Unbundle By Name(w935) -> ("Distance 2"=w934:dbl)
        n460 = call "Read Encoders.vi"("Reset"=FALSE, "Right Encoder"=w943, "Left Encoder"=w944) -> ("Encoder Values"=w932:T31, "Right Encoder Out"=w941:T27, "Left Encoder Out"=w942:T27)  [unwired: 6 in]
        n461 = Tick Count (ms)() -> (millisecond timer value=w961:u32)
        n462 = Bundle By Name(cluster=w940, "Load"=FALSE, "Shoot"=FALSE, "Elevator"=TRUE, "Two Discs"=FALSE) -> (w937:T6)
        n463 = call "AutoSpeed.vi"("Auto Speed Constants"=w957, "Encoder Values"=w932, "Two Disc Distance"=0.0, "Reinitialize"=w948, "PID settings"=w931, "Target Distance"=w934) -> ("Finish"=w954:bool, "Backward"=w953:bool, "Y axis Speed"=w955:dbl)  [unwired: 2 in, 1 out]
        n464 = call <vilib>:"WPI_GyroGetAngle.vi"("GyroDevRef"=w939) -> ("Angle"=w952:dbl, "GyroDevRef"=w938:T21)  [unwired: 7 in, 2 out]
        n465 = Subtract(x=w961, y=w933) -> (x-y=w962:u32)
        n466 = Greater Or Equal?(x=w962, y=u32 14500) -> (x >= y?=w960:bool)
        n467 = call "Auto Encoder Steering.vi"("Backward"=w953, "Gyro Angle"=w952, "Angle setpoint"=0.0) -> ("Steering"=w950:dbl)  [unwired: 7 in, 1 out]
        n468 = global write "Robot Global Data.vi" "Auton Commands"(w937) -> ()
        n469 = call-poly <vilib>:"WPI_RobotDriveArcadeDrive.vi"("Y axis value"=w955, "X axis value"=w950, "RobotDriveDevRef"=w946) -> ("RobotDriveDevRef"=w945:T7)  [unwired: 1 in, 7 out]
        n470 = Compound Arithmetic op=OR(w954, w960) -> (w949:bool)
      }
    }
  }
  n471 = disable-structure shown="Disabled" {
    frame Disabled {
      n472 = call <vilib>:"WPI_RobotDriveRefNum Registry Get.vi"("refnum name"="Left and Right Motors") -> ("RobotDriveDevRef"=w1013:T7)  [unwired: 1 in, 9 out]
      n473 = call-poly <vilib>:"WPI_RobotDriveArcadeDrive.vi"("Y axis value"=0.5 ("X axis value"), "X axis value"=0.25, "RobotDriveDevRef"=w1013) -> ("Motor Values"=w1012:dbl[], "RobotDriveDevRef"=w1016:T7)  [unwired: 1 in, 6 out]
      n474 = call <vilib>:"SD Write Numeric Array.vi"("Numeric Array"=w1012, "Name"="RobotDrive Motors") -> ()  [unwired: 8 in, 2 out]
      n475 = call <vilib>:"WPI_RobotDriveDelayAndUpdateSafety.vi"("Delay (s)"=1.0, "RobotDriveDevRef"=w1016) -> ("RobotDriveDevRef 2"=w1005:T7)  [unwired: 8 in, 1 out]
      n476 = call-poly <vilib>:"WPI_RobotDriveArcadeDrive.vi"("Y axis value"=0.5 ("X axis value"), "X axis value"=0.25, "RobotDriveDevRef"=w1005) -> ("Motor Values"=w1010:dbl[], "RobotDriveDevRef"=w1008:T7)  [unwired: 1 in, 6 out]
      n477 = call <vilib>:"SD Write Numeric Array.vi"("Numeric Array"=w1010) -> ()  [unwired: 9 in, 2 out]
      n478 = call <vilib>:"WPI_RobotDriveDelayAndUpdateSafety.vi"("Delay (s)"=1.0, "RobotDriveDevRef"=w1008) -> ()  [unwired: 8 in, 2 out]
    }
    frame Enabled {
    }
  }
  n479 = while {
    shift-right: [w1032] -> _
    shift-left: w2 -> [w1033]
    shift-right: [w1020] -> _
    shift-left: w3 -> [w1022]
    stop <- TRUE stop-if-true
    w1028 = 0.0 ("Steering")
    w1021 = 0.0 ("X axis value")
    # "Stop"
    n480 = local write "Steering"(w1028) -> ()
    n481 = call-poly <vilib>:"WPI_RobotDriveArcadeDrive.vi"("Y axis value"=w1021, "X axis value"=w1021, "RobotDriveDevRef"=w1033) -> ("Motor Values"=w1029:dbl[], "RobotDriveDevRef"=w1032:T7)  [unwired: 1 in, 6 out]
    n482 = local write "Y axis Speed"(w1028) -> ()
    n483 = call <vilib>:"SD Write Numeric Array.vi"("Numeric Array"=w1029, "Name"="RobotDrive Motors") -> ()  [unwired: 8 in, 2 out]
    n484 = Bundle By Name(cluster=w1022, "Load"=FALSE, "Shoot"=FALSE, "Low Gear"=FALSE, "Azimuth"=FALSE ("Elevator"), "Elevator"=FALSE, "Warmup"=FALSE) -> (w1020:T6)
    n485 = global write "Robot Global Data.vi" "Auton Commands"(w1020) -> ()
  }
